vi "Lab Panel V2.2.vi"() -> ()   [LabVIEW 2013]
uses:
  <vilib>/Platform/TimedLoop/XDataNode/timing_clust.ctl
  <vilib>/Platform/TimedLoop/XDataNode/nitl_modes.ctl
  <vilib>/Platform/TimedLoop/XDataNode/wakeup.ctl
  <vilib>/platform/TimedLoop/XDataNode/XDataNode.xnode
  <vilib>/Platform/TimedLoop/XDataNode/XDNodeRunTimeDep.lvlib
panel:
  out "TEMP update":bool
  out "AI update":bool
  in  "stop":bool
  in  "Tab Control 2":T1(tab)
  out "LAB05-2 (SIG)":T2 {"PF" format="%.2f"; "AMPS" format="%.1f"}
  out "LAB05-1 (SIG)":T2 {"PF" format="%.2f"; "AMPS" format="%.1f"}
  out "LAB04-2 (SIG)":T2 {"PF" format="%.2f"; "AMPS" format="%.1f"}
  out "LAB04-1 (SIG)":T2 {"PF" format="%.2f"; "AMPS" format="%.1f"}
  out "LAB03-2 (SIG)":T2 {"PF" format="%.2f"; "AMPS" format="%.1f"}
  out "LAB03-1 (SIG)":T2 {"PF" format="%.2f"; "AMPS" format="%.1f"}
  out "LAB02-2 (SIG)":T2 {"PF" format="%.2f"; "AMPS" format="%.1f"}
  in  "LAB01-1RUN":bool
  in  "LAB05-1 (O/I)":bool
  in  "LAB05-2 (O/I)":bool
  in  "LAB04-1 (O/I)":bool
  in  "LAB04-2 (O/I)":bool
  in  "LAB02-1 (O/I)":bool
  in  "LAB02-2 (O/I)":bool
  in  "LAB01-2 (O/I)":bool
  in  "LAB01-1 (O/I)":bool
  in  "LAB03-1 (O/I)":bool
  in  "LAB05-2 RUN":bool
  in  "LAB05-1 RUN":bool
  in  "LAB04-2 RUN":bool
  in  "LAB04-1 RUN":bool
  in  "LAB03-2 RUN":bool
  in  "LAB03-1 RUN":bool
  in  "LAB02-2 RUN":bool
  in  "LAB02-1 RUN":bool
  in  "LAB01-2 RUN":bool
  in  "LAB05-2 SELECT":T3(radio)
  in  "LAB05-1 SELECT":T3(radio)
  in  "LAB04-2 SELECT":T3(radio)
  in  "LAB04-1 SELECT":T3(radio)
  in  "LAB03-2 SELECT":T3(radio)
  in  "LAB03-1 SELECT":T3(radio)
  in  "LAB02-2 SELECT":T3(radio)
  in  "LAB02-1 SELECT":T3(radio)
  in  "LAB01-2 SELECT":T3(radio)
  in  "LAB01-1 SELECT":T3(radio)
  in  "LAB03-2 (O/I)":bool
  out "LAB01-1 (SIG)":T2 {"PF" format="%.2f"; "AMPS" format="%.1f"}
  out "LAB01-2 (SIG)":T2 {"PF" format="%.2f"; "AMPS" format="%.1f"}
  out "LAB02-1 (SIG)":T2 {"PF" format="%.2f"; "AMPS" format="%.1f"}
  in  "LAB05 (SETTINGS 1)":T4={"1 Name"="", "1 Description"="", "1 (CYCLES)"=1.0, "1 (T-RISE mins)"=1.0, "1 (T-RISE deg C)"=1.0, "2 Name"="", "2 Description"="", "2 (CYCLES)"=1.0, "2 (T-RISE mins)"=1.0, "2 (T-RISE deg C)"=1.0} {"2 (T-RISE deg C)" min=1.0 max=100.0 step=1.0 format="%#.0f"; "2 (T-RISE mins)" min=0.0 max=1000.0 step=10.0 format="%#.0f"; "2 (CYCLES)" min=0.0 max=100000.0 step=10.0; "1 (T-RISE deg C)" min=1.0 max=100.0 step=1.0 format="%#.0f"; "1 (T-RISE mins)" min=0.0 max=1000.0 step=10.0 format="%#.0f"; "1 (CYCLES)" min=0.0 max=100000.0 step=10.0}
  in  "LAB04 (SETTINGS 1)":T4={"1 Name"="", "1 Description"="", "1 (CYCLES)"=1.0, "1 (T-RISE mins)"=1.0, "1 (T-RISE deg C)"=1.0, "2 Name"="", "2 Description"="", "2 (CYCLES)"=1.0, "2 (T-RISE mins)"=1.0, "2 (T-RISE deg C)"=1.0} {"2 (T-RISE deg C)" min=1.0 max=100.0 step=1.0 format="%#.0f"; "2 (T-RISE mins)" min=0.0 max=1000.0 step=10.0 format="%#.0f"; "2 (CYCLES)" min=0.0 max=100000.0 step=10.0; "1 (T-RISE deg C)" min=1.0 max=100.0 step=1.0 format="%#.0f"; "1 (T-RISE mins)" min=0.0 max=1000.0 step=10.0 format="%#.0f"; "1 (CYCLES)" min=0.0 max=100000.0 step=10.0}
  in  "LAB03 (SETTINGS 1)":T4={"1 Name"="", "1 Description"="", "1 (CYCLES)"=1.0, "1 (T-RISE mins)"=1.0, "1 (T-RISE deg C)"=1.0, "2 Name"="", "2 Description"="", "2 (CYCLES)"=1.0, "2 (T-RISE mins)"=1.0, "2 (T-RISE deg C)"=1.0} {"2 (T-RISE deg C)" min=1.0 max=100.0 step=1.0 format="%#.0f"; "2 (T-RISE mins)" min=0.0 max=1000.0 step=10.0 format="%#.0f"; "2 (CYCLES)" min=0.0 max=100000.0 step=10.0; "1 (T-RISE deg C)" min=1.0 max=100.0 step=1.0 format="%#.0f"; "1 (T-RISE mins)" min=0.0 max=1000.0 step=10.0 format="%#.0f"; "1 (CYCLES)" min=0.0 max=100000.0 step=10.0}
  out "LAB05 (DISP 1)":T5 {"2 (T-RISE min)" format="%#.0f"; "2 (CYCLE)" format="%#.0f"; "1 (T-RISE min)" format="%#.0f"; "1 (CYCLE)" format="%#.0f"}
  out "LAB04 (DISP 1)":T5 {"2 (T-RISE min)" format="%#.0f"; "2 (CYCLE)" format="%#.0f"; "1 (T-RISE min)" format="%#.0f"; "1 (CYCLE)" format="%#.0f"}
  out "LAB03 (DISP 1)":T5 {"2 (T-RISE min)" format="%#.0f"; "2 (CYCLE)" format="%#.0f"; "1 (T-RISE min)" format="%#.0f"; "1 (CYCLE)" format="%#.0f"}
  out "LAB02 (DISP 1)":T5 {"2 (T-RISE min)" format="%#.0f"; "2 (CYCLE)" format="%#.0f"; "1 (T-RISE min)" format="%#.0f"; "1 (CYCLE)" format="%#.0f"}
  in  "LAB02 (SETTINGS 1)":T4={"1 Name"="", "1 Description"="", "1 (CYCLES)"=1.0, "1 (T-RISE mins)"=1.0, "1 (T-RISE deg C)"=1.0, "2 Name"="", "2 Description"="", "2 (CYCLES)"=1.0, "2 (T-RISE mins)"=1.0, "2 (T-RISE deg C)"=1.0} {"2 (T-RISE deg C)" min=1.0 max=100.0 step=1.0 format="%#.0f"; "2 (T-RISE mins)" min=0.0 max=1000.0 step=10.0 format="%#.0f"; "2 (CYCLES)" min=0.0 max=100000.0 step=10.0; "1 (T-RISE deg C)" min=1.0 max=100.0 step=1.0 format="%#.0f"; "1 (T-RISE mins)" min=0.0 max=1000.0 step=10.0 format="%#.0f"; "1 (CYCLES)" min=0.0 max=100000.0 step=10.0}
  out "LAB01 (DISP 1)":T5 {"2 (T-RISE min)" format="%#.0f"; "2 (CYCLE)" format="%#.0f"; "1 (T-RISE min)" format="%#.0f"; "1 (CYCLE)" format="%#.0f"}
  in  "LAB01 (SETTINGS 1)":T4={"1 Name"="", "1 Description"="", "1 (CYCLES)"=1.0, "1 (T-RISE mins)"=1.0, "1 (T-RISE deg C)"=1.0, "2 Name"="", "2 Description"="", "2 (CYCLES)"=1.0, "2 (T-RISE mins)"=1.0, "2 (T-RISE deg C)"=1.0} {"2 (T-RISE deg C)" min=1.0 max=100.0 step=1.0 format="%#.0f"; "2 (T-RISE mins)" min=0.0 max=1000.0 step=10.0 format="%#.0f"; "2 (CYCLES)" min=0.0 max=100000.0 step=10.0; "1 (T-RISE deg C)" min=1.0 max=100.0 step=1.0 format="%#.0f"; "1 (T-RISE mins)" min=0.0 max=1000.0 step=10.0 format="%#.0f"; "1 (CYCLES)" min=0.0 max=100000.0 step=10.0}
  in  "JIG ON TIME (S)":dbl=1.0 min=1.0 max=10.0 step=0.5 format="%.1g"
  in  "JIG OFF TIME (S)":dbl=2.0 min=2.0 max=10.0 step=0.5 format="%.1g"
  out "LAB01-1 (JIG)":bool
  out "LAB01-2 (JIG)":bool
  out "LAB02-1 (JIG)":bool
  out "LAB02-2 (JIG)":bool
  out "LAB03-1 (JIG)":bool
  out "LAB03-2 (JIG)":bool
  out "LAB04-1 (JIG)":bool
  out "LAB04-2 (JIG)":bool
  out "LAB05-1 (JIG)":bool
  out "LAB05-2 (JIG)":bool
  in  "Tab Control":T6(tab)
  out "LAB01-2 (GRAPH)":dynamicdata(graph)
  out "LAB01-1 (GRAPH)":dynamicdata(graph)
  out "LAB02-2 (GRAPH)":dynamicdata(graph)
  out "LAB02-1 (GRAPH)":dynamicdata(graph)
  out "LAB03-2 (GRAPH)":dynamicdata(graph)
  out "LAB03-1 (GRAPH)":dynamicdata(graph)
  out "LAB04-2 (GRAPH)":dynamicdata(graph)
  out "LAB04-1 (GRAPH)":dynamicdata(graph)
  out "LAB05-2 (GRAPH)":dynamicdata(graph)
  out "LAB05-1 (GRAPH)":dynamicdata(graph)
  out "LAB05 TEMP":T7
  out "LAB04 TEMP":T7
  out "LAB02 TEMP":T7
  out "LAB01 TEMP":T7
  out "LAB03 TEMP":T7
  out "Analog Error Array":errorcluster[](array[cluster])
  out "AI loop time":dbl format="%.6g"
  out "loops":dbl
  in  "loop  delay(mS)":dbl
  out "on loops":dbl
  out "off loops":dbl
  out "jig cycle":dbl
  out "LAB01-1 (TDMS)":refnum<k34>
  out "LAB01-2 (TDMS)":refnum<k34>
  out "data file error":errorcluster
  out "LAB01 (CAL)":T8 {"2 (TN) cal" min=0.0 step=0.01 format="%.2f"; "2 (TL) cal" min=0.0 step=0.01 format="%.2f"; "2 (PF) cal" min=0.0 step=0.01 format="%.2f"; "2 (V) cal" min=0.0 step=0.01 format="%.2f"; "2 (A) cal" min=0.0 step=0.01 format="%.2f"; "1 (TN) cal" min=0.0 step=0.01 format="%.2f"; "1 (TL) cal" min=0.0 step=0.01 format="%.2f"; "1 (PF) cal" min=0.0 step=0.01 format="%.2f"; "1 (V) cal" min=0.0 step=0.01 format="%.2f"; "1  (A) cal" min=0.0 step=0.01 format="%.2f"}
  out "LAB03 (CAL)":T8 {"2 (TN) cal" min=0.0 step=0.01 format="%.2f"; "2 (TL) cal" min=0.0 step=0.01 format="%.2f"; "2 (PF) cal" min=0.0 step=0.01 format="%.2f"; "2 (V) cal" min=0.0 step=0.01 format="%.2f"; "2 (A) cal" min=0.0 step=0.01 format="%.2f"; "1 (TN) cal" min=0.0 step=0.01 format="%.2f"; "1 (TL) cal" min=0.0 step=0.01 format="%.2f"; "1 (PF) cal" min=0.0 step=0.01 format="%.2f"; "1 (V) cal" min=0.0 step=0.01 format="%.2f"; "1  (A) cal" min=0.0 step=0.01 format="%.2f"}
  out "LAB02 (CAL)":T9 {"2 (TN) cal" min=0.0 step=0.01 format="%.2f"; "2 (TL) cal" min=0.0 step=0.01 format="%.2f"; "2 (PF) cal" min=0.0 step=0.01 format="%.2f"; "2 (V) cal" min=0.0 step=0.01 format="%.2f"; "2 (A) cal" min=0.0 step=0.01 format="%.2f"; "1 (TN) cal" min=0.0 step=0.01 format="%.2f"; "1 (TL) cal" min=0.0 step=0.01 format="%.2f"; "1 (PF) cal" min=0.0 step=0.01 format="%.2f"; "1 (V) cal" min=0.0 step=0.01 format="%.2f"; "1 (A) cal" min=0.0 step=0.01 format="%.2f"}
  out "LAB05 (CAL)":T8 {"2 (TN) cal" min=0.0 step=0.01 format="%.2f"; "2 (TL) cal" min=0.0 step=0.01 format="%.2f"; "2 (PF) cal" min=0.0 step=0.01 format="%.2f"; "2 (V) cal" min=0.0 step=0.01 format="%.2f"; "2 (A) cal" min=0.0 step=0.01 format="%.2f"; "1 (TN) cal" min=0.0 step=0.01 format="%.2f"; "1 (TL) cal" min=0.0 step=0.01 format="%.2f"; "1 (PF) cal" min=0.0 step=0.01 format="%.2f"; "1 (V) cal" min=0.0 step=0.01 format="%.2f"; "1  (A) cal" min=0.0 step=0.01 format="%.2f"}
  out "LAB04 (CAL)":T8 {"2 (TN) cal" min=0.0 step=0.01 format="%.2f"; "2 (TL) cal" min=0.0 step=0.01 format="%.2f"; "2 (PF) cal" min=0.0 step=0.01 format="%.2f"; "2 (V) cal" min=0.0 step=0.01 format="%.2f"; "2 (A) cal" min=0.0 step=0.01 format="%.2f"; "1 (TN) cal" min=0.0 step=0.01 format="%.2f"; "1 (TL) cal" min=0.0 step=0.01 format="%.2f"; "1 (PF) cal" min=0.0 step=0.01 format="%.2f"; "1 (V) cal" min=0.0 step=0.01 format="%.2f"; "1  (A) cal" min=0.0 step=0.01 format="%.2f"}
  out "calibration file error out":errorcluster
  in  "CALIBRATE":bool
  # "LAB01"
  # "LAB02"
  # "LAB05"
  # "LAB03"
  # "LAB04"
  # "LAB01"
  # "LAB02"
  # "LAB03"
  # "LAB04"
  # "LAB05"
  # "JIG SET"
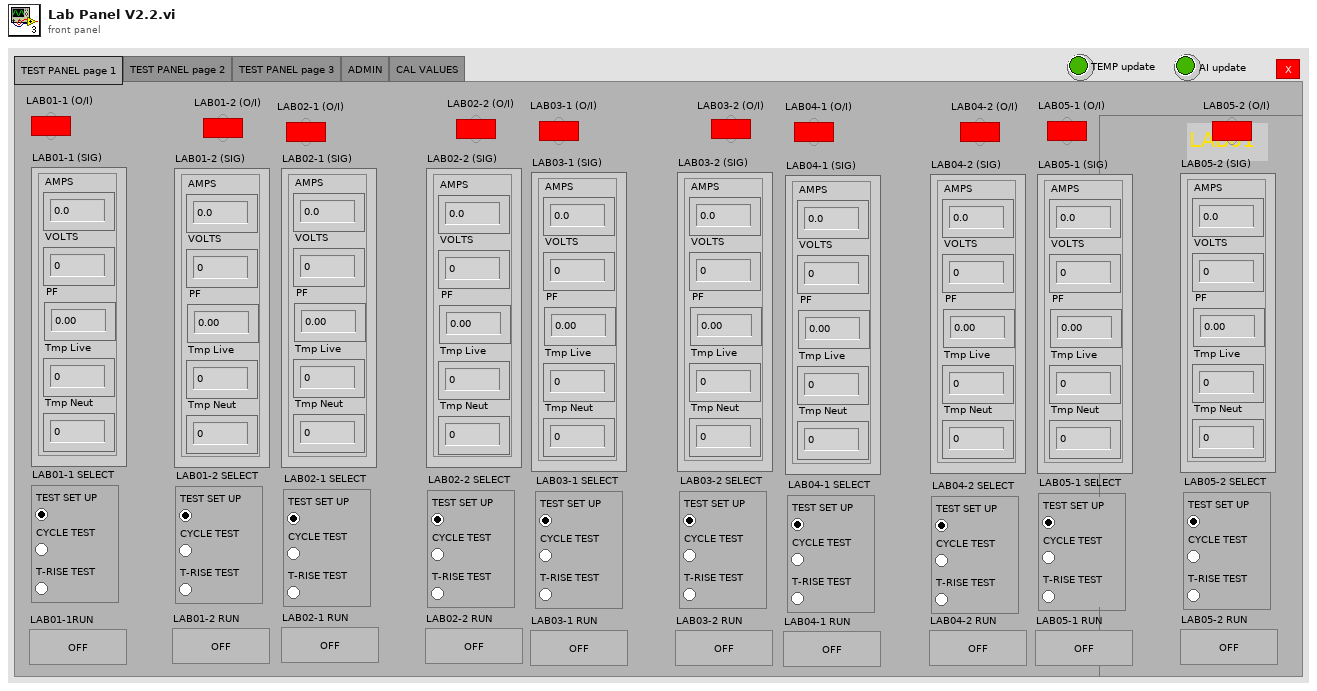
[diagram p1: front panel]
types:
  T1 = enum32{"TEST PANEL page 1", "TEST PANEL page 2", "TEST PANEL page 3", "ADMIN", "CAL VALUES"}
  T2 = cluster{"AMPS":dbl, "VOLTS":dbl, "PF":dbl, "Tmp Live":dbl, "Tmp Neut":dbl}
  T3 = enum32{"TEST SET UP", "CYCLE TEST", "T-RISE TEST"}
  T4 = cluster{"1 Name":string, "1 Description":string, "1 (CYCLES)":dbl, "1 (T-RISE mins)":dbl, "1 (T-RISE deg C)":dbl, "2 Name":string, "2 Description":string, "2 (CYCLES)":dbl, "2 (T-RISE mins)":dbl, "2 (T-RISE deg C)":dbl}
  T5 = cluster{"1 (CYCLE)":dbl, "1 (T-RISE min)":dbl, "1 (STATUS)":string, "2 (CYCLE)":dbl, "2 (T-RISE min)":dbl, "2 (STATUS)":string}
  T6 = enum32{"LAB01", "LAB02", "LAB03", "LAB04", "LAB05", "TEMPERATURE", "ERROR"}
  T7 = cluster{"T1 Live":dbl, "T1 Neut":dbl, "T2 Live":dbl, "T2 Neut":dbl, "ID":dbl, "ER":dbl}
  T8 = cluster{"1  (A) cal":dbl, "1 (V) cal":dbl, "1 (PF) cal":dbl, "1 (TL) cal":dbl, "1 (TN) cal":dbl, "2 (A) cal":dbl, "2 (V) cal":dbl, "2 (PF) cal":dbl, "2 (TL) cal":dbl, "2 (TN) cal":dbl}
  T9 = cluster{"1 (A) cal":dbl, "1 (V) cal":dbl, "1 (PF) cal":dbl, "1 (TL) cal":dbl, "1 (TN) cal":dbl, "2 (A) cal":dbl, "2 (V) cal":dbl, "2 (PF) cal":dbl, "2 (TL) cal":dbl, "2 (TN) cal":dbl}
  T10 = typedef "XDNodeRunTimeDep.lvlib/timing_clust.ctl" = cluster{"Expected End [f-1]":u64, "Actual End [f-1]":u64, "Finished Late? [f-1]":bool, "Expected End [i-1]":u64, "Actual End [i-1]":u64, "Finished Late? [i-1]":bool, "Expected Start [i]":u64, "Actual Start [i]":u64, "Expected Start [f]":u64, "Actual Start [f]":u64, "Source Name":string, "Structure Name":string, "Period":i64, "Deadline":i64, "Offset":i64, "Start":i64, "Priority":i32, "Timeout":i32, "Mode":T11, "Wakeup Reason":T12, "Error":errorcluster, "Source Type":string, "Secondary Source Type":string, "Global End Time":u64, "Global Start Time":u64, "Frame Duration":u64, "Iteration Duration":u64, "Assigned CPU":i32, "I/O Scan Engine Mode":u32}
  T11 = typedef "XDNodeRunTimeDep.lvlib/nitl_modes.ctl" = enum32{"No Change", "Process missed periods, maintain original phase", "Discard missed periods, maintain original phase", "Process missed periods, ignore original phase", "Discard missed periods, ignore original phase"}
  T12 = typedef "XDNodeRunTimeDep.lvlib/wakeup.ctl" = enum32{"Normal", "Aborted", "Asynchronous wakeup", "Timing source error", "Timed loop error", "Timeout"}
  T13 = enum16{"open", "open or create", "create or replace", "create", "open (read-only)"}
  T14 = cluster{"T1":dbl, "T2":dbl, "T3":dbl, "T4":dbl, "ID":dbl, "ER":dbl}
  T15 = cluster{"LAB01-1 (A)":dbl, "LAB01-1 (V)":dbl, "LAB01-1 (PF)":dbl, "LAB01-2 (A)":dbl, "LAB01-2 (V)":dbl, "LAB01-2 (PF)":dbl}
  T16 = cluster{"LAB02-1 (A)":dbl, "LAB02-1 (V)":dbl, "LAB02-1 (PF)":dbl, "LAB02-2 (A)":dbl, "LAB02-2 (V)":dbl, "LAB02-2 (PF)":dbl}
  T17 = cluster{"LAB03-1 (A)":dbl, "LAB03-1 (V)":dbl, "LAB03-1 (PF)":dbl, "LAB03-2 (A)":dbl, "LAB03-2 (V)":dbl, "LAB03-2 (PF)":dbl}
  T18 = cluster{"LAB04-1 (A)":dbl, "LAB04-1 (V)":dbl, "LAB04-1 (PF)":dbl, "LAB04-2 (A)":dbl, "LAB04-2 (V)":dbl, "LAB04-2 (PF)":dbl}
  T19 = cluster{"LAB05-1 (A)":dbl, "LAB05-1 (V)":dbl, "LAB05-1 (PF)":dbl, "LAB05-2 (A)":dbl, "LAB05-2 (V)":dbl, "LAB05-2 (PF)":dbl}
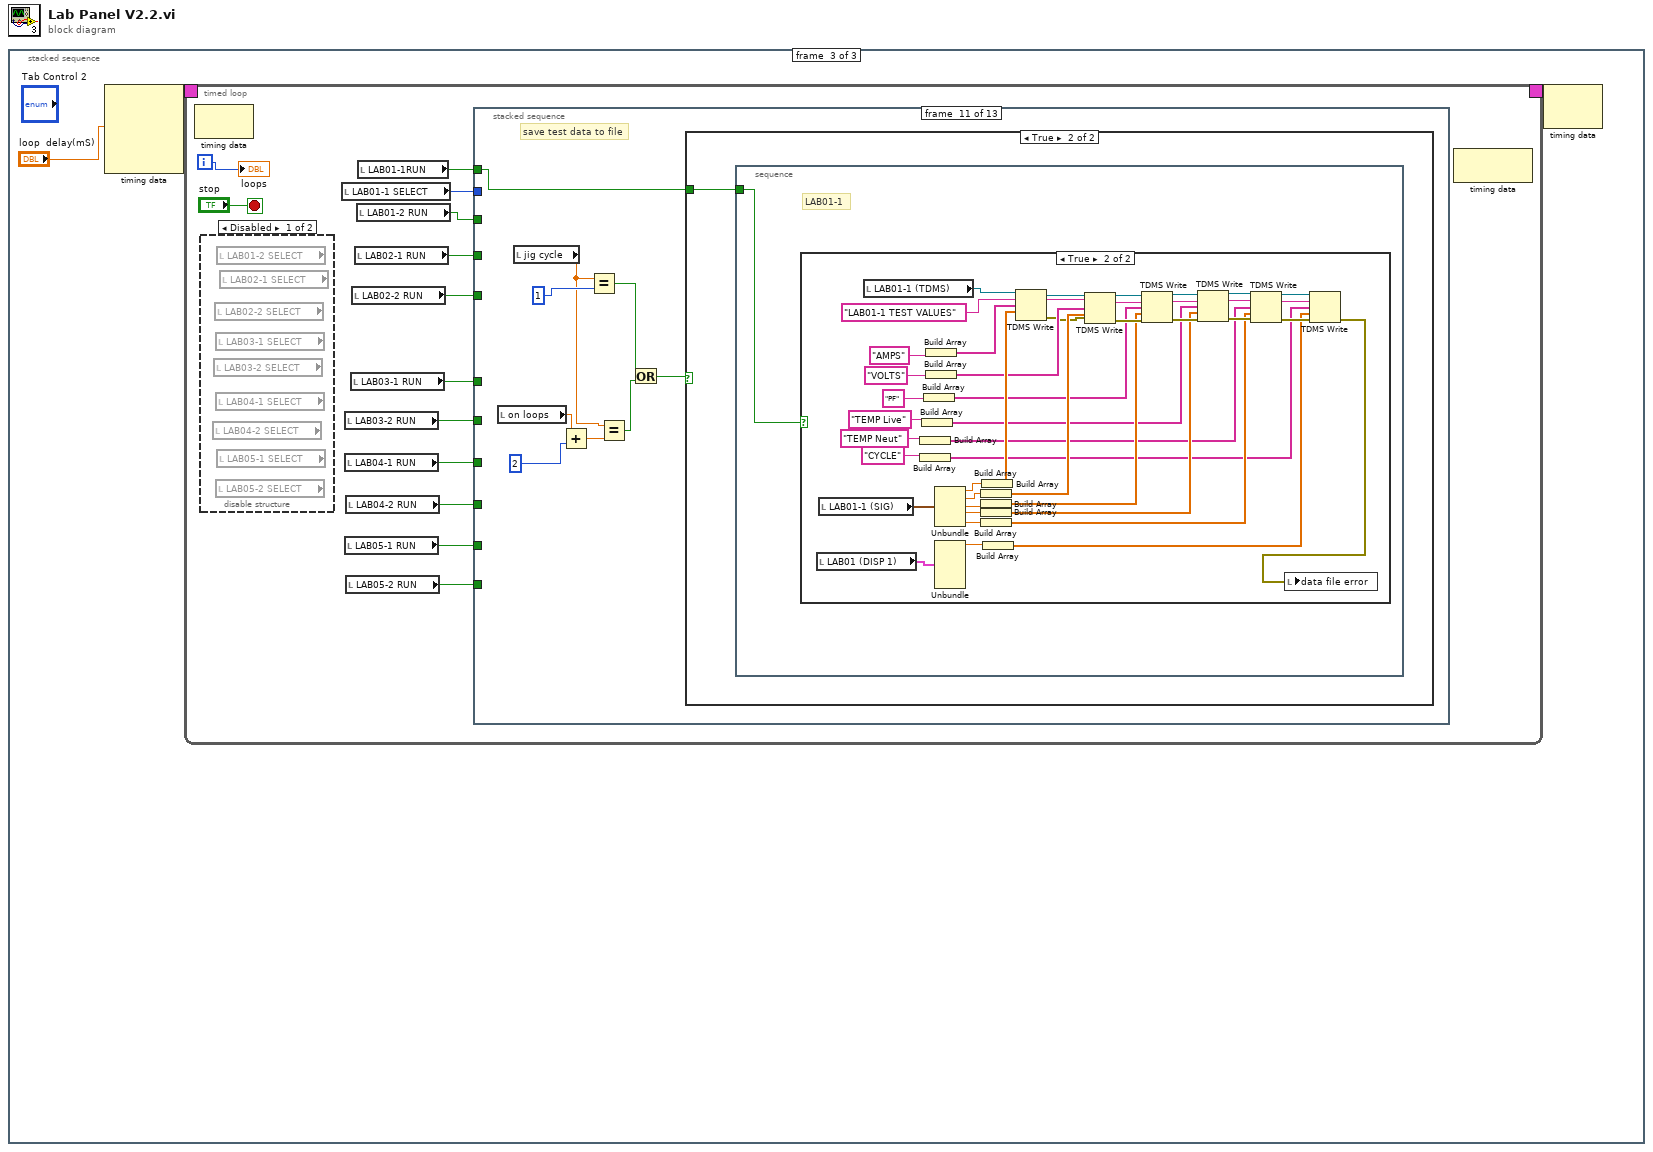
[diagram p0: block diagram]
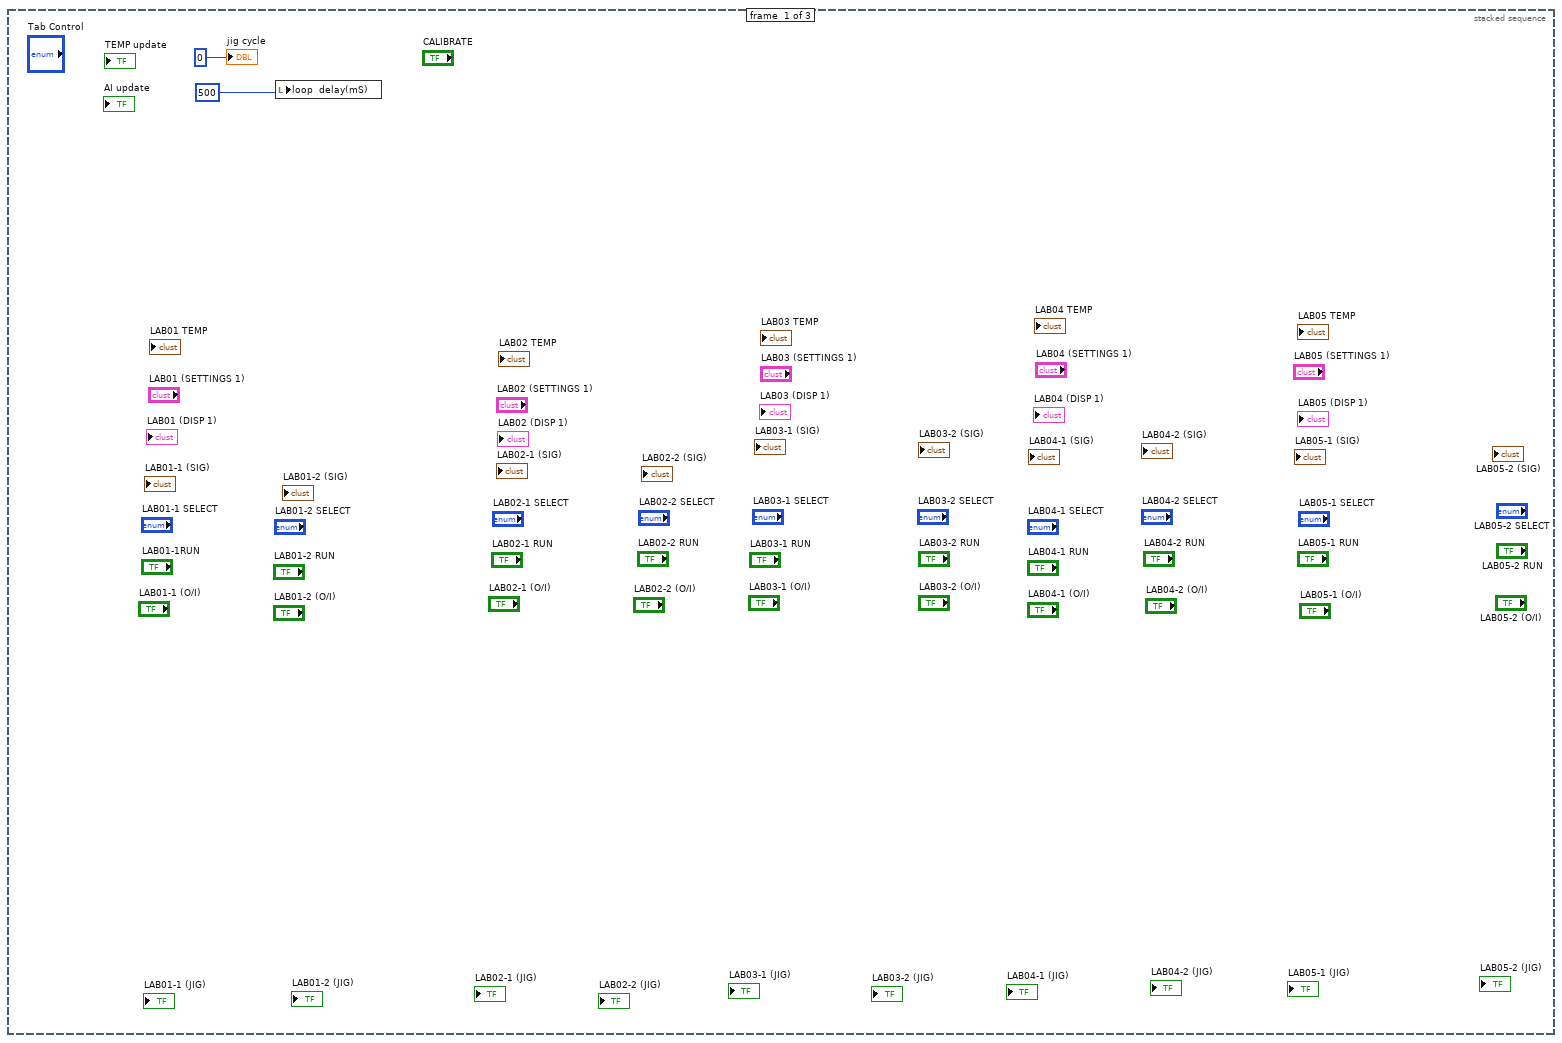
[diagram p2: hidden frame]
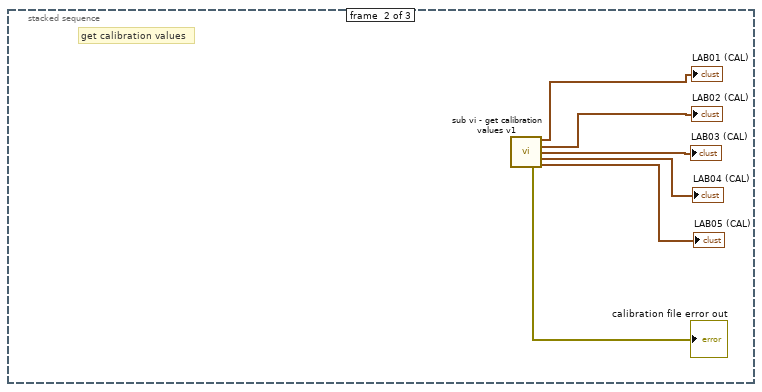
[diagram p3: hidden frame]
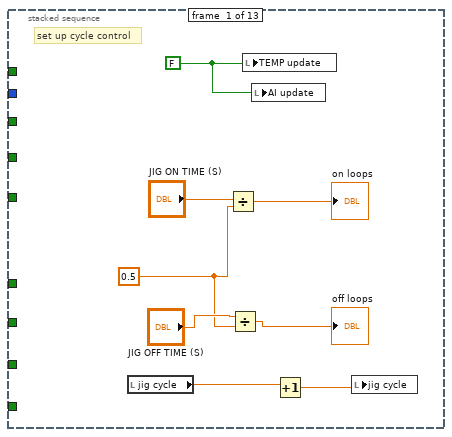
[diagram p5: hidden frame]
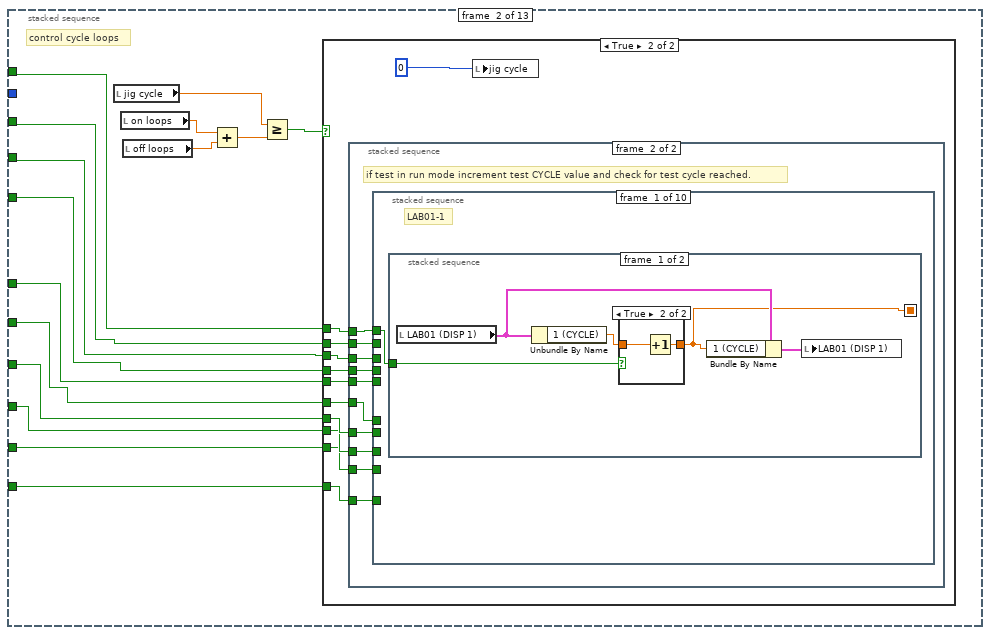
[diagram p6: hidden frame]
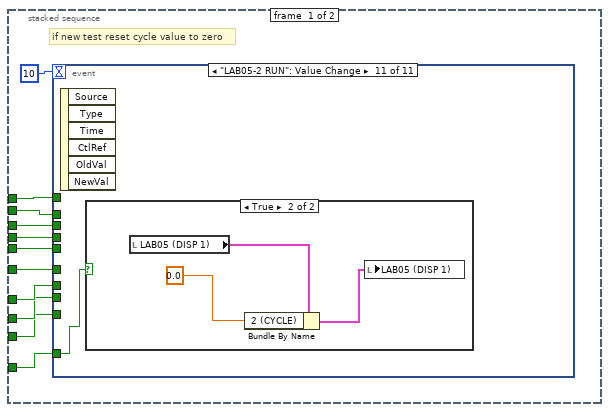
[diagram p8: hidden frame]
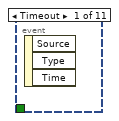
[diagram p9: hidden frame]
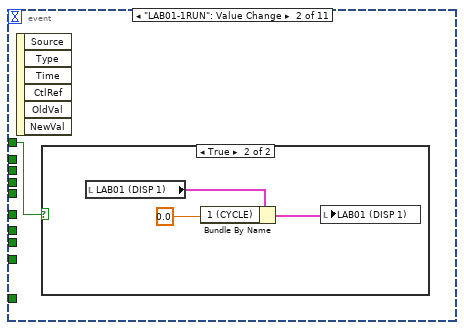
[diagram p10: hidden frame]
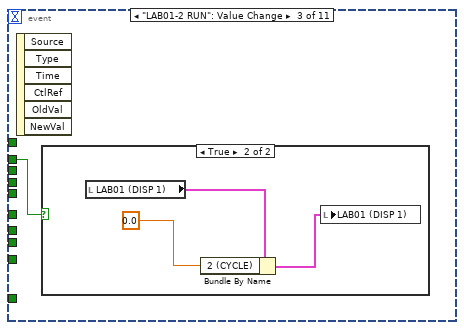
[diagram p12: hidden frame]
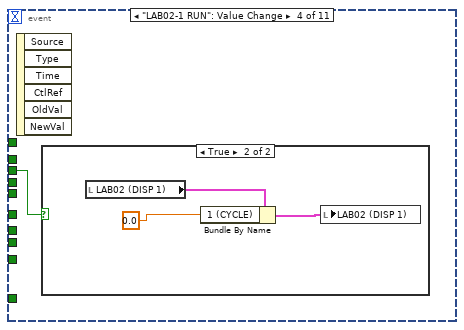
[diagram p14: hidden frame]
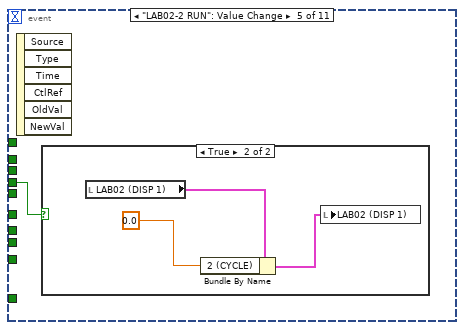
[diagram p16: hidden frame]
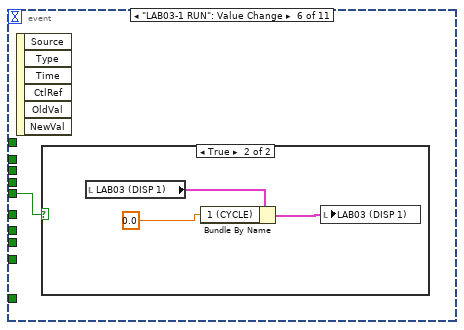
[diagram p18: hidden frame]
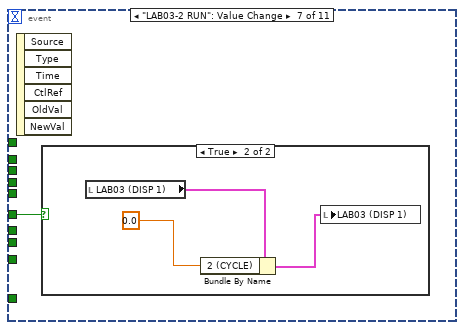
[diagram p20: hidden frame]
diagram:
  n1 = stacked-sequence {
    frame #0 {
      n2 = local write "loop  delay(mS)"(500) -> ()
      "jig cycle" <- 0
    }
    frame #1 {
      # "get calibration values"
      n3 = call "sub vi - get calibration values v1.vi"() -> ("LAB01 (CAL)"=→"LAB01 (CAL)":T8, "LAB02 (CAL)"=→"LAB02 (CAL)":T9, "LAB03 (CAL)"=→"LAB03 (CAL)":T8, "LAB04 (CAL)"=→"LAB04 (CAL)":T8, "calibration file error out"=→"calibration file error out":errorcluster, "LAB05 (CAL)"=→"LAB05 (CAL)":T8)  [unwired: 10 in]
    }
    frame #2 {
      n4 = node-c288("loop  delay(mS)") -> (w11:T10)  [unwired: 3 in]
      n5 = timed-loop {
        timing: w11 -> [_]
        timing-out: [_] -> w10
        i -> [w24]
        stop <- "stop" stop-if-true
        n6 = node-c288() -> ()  [unwired: 1 in, 1 out]
        n7 = disable-structure shown="Disabled" {
          frame Disabled {
            n8 = local read "LAB04-2 SELECT"() -> ()  [unwired: 1 out]
            n9 = local read "LAB03-2 SELECT"() -> ()  [unwired: 1 out]
            n10 = local read "LAB02-2 SELECT"() -> ()  [unwired: 1 out]
            n11 = local read "LAB03-1 SELECT"() -> ()  [unwired: 1 out]
            n12 = local read "LAB04-1 SELECT"() -> ()  [unwired: 1 out]
            n13 = local read "LAB05-2 SELECT"() -> ()  [unwired: 1 out]
            n14 = local read "LAB01-2 SELECT"() -> ()  [unwired: 1 out]
            n15 = local read "LAB05-1 SELECT"() -> ()  [unwired: 1 out]
            n16 = local read "LAB02-1 SELECT"() -> ()  [unwired: 1 out]
          }
          frame Enabled {
          }
        }
        n17 = local read "LAB01-1 SELECT"() -> (w12:T3)
        n18 = local read "LAB03-2 RUN"() -> (w17:bool)
        n19 = local read "LAB04-1 RUN"() -> (w16:bool)
        n20 = local read "LAB05-1 RUN"() -> (w14:bool)
        n21 = local read "LAB04-2 RUN"() -> (w15:bool)
        n22 = local read "LAB05-2 RUN"() -> (w13:bool)
        n23 = local read "LAB03-1 RUN"() -> (w18:bool)
        n24 = local read "LAB02-2 RUN"() -> (w19:bool)
        n25 = local read "LAB02-1 RUN"() -> (w20:bool)
        n26 = local read "LAB01-2 RUN"() -> (w21:bool)
        n27 = local read "LAB01-1RUN"() -> (w22:bool)
        n28 = stacked-sequence {
          tunnel: w22 -> [_ w44 w336 _ w411 w466 _ _ _ _ w833 _ _]
          tunnel: w21 -> [_ w43 w335 _ _ _ _ _ _ _ _ _ _]
          tunnel: w20 -> [_ w42 w334 _ _ _ _ _ _ _ _ _ _]
          tunnel: w19 -> [_ w41 w333 _ _ _ _ _ _ _ _ _ _]
          tunnel: w18 -> [_ w40 w332 _ _ _ _ _ _ _ _ _ _]
          tunnel: w17 -> [_ w39 w331 _ _ _ _ _ _ _ _ _ _]
          tunnel: w16 -> [_ w38 w330 _ _ _ _ _ _ _ _ _ _]
          tunnel: w15 -> [_ w37 w329 _ _ _ _ _ _ _ _ _ _]
          tunnel: w14 -> [_ w36 w328 _ _ _ _ _ _ _ _ _ _]
          tunnel: w13 -> [_ w35 w327 _ _ _ _ _ _ _ _ _ _]
          tunnel: w12 -> [_ _ _ _ w412 _ _ _ _ _ _ _ _]
          frame #0 {
            w27 = FALSE
            w32 = 0.5
            # "set up cycle control"
            n29 = local read "jig cycle"() -> (w31:dbl)
            n30 = Divide(x="JIG ON TIME (S)", y=w32) -> (x/y=→"on loops":dbl)
            n31 = Divide(x="JIG OFF TIME (S)", y=w32) -> (x/y=→"off loops":dbl)
            n32 = local write "TEMP update"(w27) -> ()
            n33 = local write "AI update"(w27) -> ()
            n34 = Increment(x=w31) -> (x+1=w30:dbl)
            n35 = local write "jig cycle"(w30) -> ()
          }
          frame #1 {
            # "control cycle loops"
            n36 = local read "jig cycle"() -> (w46:dbl)
            n37 = local read "on loops"() -> (w49:dbl)
            n38 = local read "off loops"() -> (w48:dbl)
            n39 = Add(x=w49, y=w48) -> (x+y=w47:dbl)
            n40 = Greater Or Equal?(x=w46, y=w47) -> (x >= y?=w45:bool)
            n41 = case shown="True" w45 {
              tunnel: w44 -> [_ w59]
              tunnel: w43 -> [_ w58]
              tunnel: w42 -> [_ w57]
              tunnel: w41 -> [_ w56]
              tunnel: w40 -> [_ w55]
              tunnel: w39 -> [_ w54]
              tunnel: w38 -> [_ w53]
              tunnel: w37 -> [_ w52]
              tunnel: w36 -> [_ w51]
              tunnel: w35 -> [_ w50]
              frame False {
              }
              frame True {
                n42 = stacked-sequence {
                  tunnel: w59 -> [w70 w121]
                  tunnel: w58 -> [w69 w120]
                  tunnel: w57 -> [w68 w119]
                  tunnel: w56 -> [w67 w118]
                  tunnel: w55 -> [w66 w117]
                  tunnel: w54 -> [w65 w116]
                  tunnel: w53 -> [w64 w115]
                  tunnel: w52 -> [w63 w114]
                  tunnel: w51 -> [w62 w113]
                  tunnel: w50 -> [w61 w112]
                  frame #0 {
                    # "if new test reset cycle value to zero"
                    n43 = event shown="[10] \"LAB05-2 RUN\": Value Change" {
                      selector: _ -> [_ _ _ _ _ _ _ _ _ _ _]
                      dyn-events: _ -> [_ _ _ _ _ _ _ _ _ _ _]
                      timeout: 10 -> [_ _ _ _ _ _ _ _ _ _ _]
                      tunnel: w70 -> [_ w72 _ _ _ _ _ _ _ _ _]
                      tunnel: w69 -> [_ _ w76 _ _ _ _ _ _ _ _]
                      tunnel: w68 -> [_ _ _ w80 _ _ _ _ _ _ _]
                      tunnel: w67 -> [_ _ _ _ w84 _ _ _ _ _ _]
                      tunnel: w66 -> [_ _ _ _ _ w88 _ _ _ _ _]
                      tunnel: w65 -> [_ _ _ _ _ _ w92 _ _ _ _]
                      tunnel: w64 -> [_ _ _ _ _ _ _ w96 _ _ _]
                      tunnel: w63 -> [_ _ _ _ _ _ _ _ w100 _ _]
                      tunnel: w62 -> [_ _ _ _ _ _ _ _ _ w104 _]
                      tunnel: w61 -> [_ _ _ _ _ _ _ _ _ _ w108]
                      event Timeout {
                        n44 = event-data() -> ()  [unwired: 1 in, 3 out]
                      }
                      event "LAB01-1RUN": Value Change {
                        n45 = event-data() -> ()  [unwired: 1 in, 6 out]
                        n46 = case shown="True" w72 {
                          frame False {
                          }
                          frame True {
                            n47 = local read "LAB01 (DISP 1)"() -> (w75:T5)
                            n48 = Bundle By Name(cluster=w75, "1 (CYCLE)"=0.0) -> (w73:T5)
                            n49 = local write "LAB01 (DISP 1)"(w73) -> ()
                          }
                        }
                      }
                      event "LAB01-2 RUN": Value Change {
                        n50 = event-data() -> ()  [unwired: 1 in, 6 out]
                        n51 = case shown="True" w76 {
                          frame False {
                          }
                          frame True {
                            n52 = local read "LAB01 (DISP 1)"() -> (w79:T5)
                            n53 = Bundle By Name(cluster=w79, "2 (CYCLE)"=0.0) -> (w78:T5)
                            n54 = local write "LAB01 (DISP 1)"(w78) -> ()
                          }
                        }
                      }
                      event "LAB02-1 RUN": Value Change {
                        n55 = event-data() -> ()  [unwired: 1 in, 6 out]
                        n56 = case shown="True" w80 {
                          frame False {
                          }
                          frame True {
                            n57 = local read "LAB02 (DISP 1)"() -> (w83:T5)
                            n58 = Bundle By Name(cluster=w83, "1 (CYCLE)"=0.0) -> (w82:T5)
                            n59 = local write "LAB02 (DISP 1)"(w82) -> ()
                          }
                        }
                      }
                      event "LAB02-2 RUN": Value Change {
                        n60 = event-data() -> ()  [unwired: 1 in, 6 out]
                        n61 = case shown="True" w84 {
                          frame False {
                          }
                          frame True {
                            n62 = local read "LAB02 (DISP 1)"() -> (w87:T5)
                            n63 = Bundle By Name(cluster=w87, "2 (CYCLE)"=0.0) -> (w86:T5)
                            n64 = local write "LAB02 (DISP 1)"(w86) -> ()
                          }
                        }
                      }
                      event "LAB03-1 RUN": Value Change {
                        n65 = event-data() -> ()  [unwired: 1 in, 6 out]
                        n66 = case shown="True" w88 {
                          frame False {
                          }
                          frame True {
                            n67 = local read "LAB03 (DISP 1)"() -> (w91:T5)
                            n68 = Bundle By Name(cluster=w91, "1 (CYCLE)"=0.0) -> (w90:T5)
                            n69 = local write "LAB03 (DISP 1)"(w90) -> ()
                          }
                        }
                      }
                      event "LAB03-2 RUN": Value Change {
                        n70 = event-data() -> ()  [unwired: 1 in, 6 out]
                        n71 = case shown="True" w92 {
                          frame False {
                          }
                          frame True {
                            n72 = local read "LAB03 (DISP 1)"() -> (w95:T5)
                            n73 = Bundle By Name(cluster=w95, "2 (CYCLE)"=0.0) -> (w94:T5)
                            n74 = local write "LAB03 (DISP 1)"(w94) -> ()
                          }
                        }
                      }
                      event "LAB04-1 RUN": Value Change {
                        n75 = event-data() -> ()  [unwired: 1 in, 6 out]
                        n76 = case shown="True" w96 {
                          frame False {
                          }
                          frame True {
                            n77 = local read "LAB04 (DISP 1)"() -> (w99:T5)
                            n78 = Bundle By Name(cluster=w99, "1 (CYCLE)"=0.0) -> (w98:T5)
                            n79 = local write "LAB04 (DISP 1)"(w98) -> ()
                          }
                        }
                      }
                      event "LAB04-2 RUN": Value Change {
                        n80 = event-data() -> ()  [unwired: 1 in, 6 out]
                        n81 = case shown="True" w100 {
                          frame False {
                          }
                          frame True {
                            n82 = local read "LAB04 (DISP 1)"() -> (w103:T5)
                            n83 = Bundle By Name(cluster=w103, "2 (CYCLE)"=0.0) -> (w102:T5)
                            n84 = local write "LAB04 (DISP 1)"(w102) -> ()
                          }
                        }
                      }
                      event "LAB05-1 RUN": Value Change {
                        n85 = event-data() -> ()  [unwired: 1 in, 6 out]
                        n86 = case shown="True" w104 {
                          frame False {
                          }
                          frame True {
                            n87 = local read "LAB05 (DISP 1)"() -> (w107:T5)
                            n88 = Bundle By Name(cluster=w107, "1 (CYCLE)"=0.0) -> (w106:T5)
                            n89 = local write "LAB05 (DISP 1)"(w106) -> ()
                          }
                        }
                      }
                      event "LAB05-2 RUN": Value Change {
                        n90 = event-data() -> ()  [unwired: 1 in, 6 out]
                        n91 = case shown="True" w108 {
                          frame False {
                          }
                          frame True {
                            n92 = local read "LAB05 (DISP 1)"() -> (w111:T5)
                            n93 = Bundle By Name(cluster=w111, "2 (CYCLE)"=0.0) -> (w110:T5)
                            n94 = local write "LAB05 (DISP 1)"(w110) -> ()
                          }
                        }
                      }
                    }
                  }
                  frame #1 {
                    # "if test in run mode increment test CYCLE value and check for test cycle reached."
                    n95 = stacked-sequence {
                      tunnel: w121 -> [w122 w139 w157 w176 w196 w217 w239 w262 w286 w311]
                      tunnel: w120 -> [_ w138 w156 w175 w195 w216 w238 w261 w285 w310]
                      tunnel: w119 -> [_ _ w155 w174 w194 w215 w237 w260 w284 w309]
                      tunnel: w118 -> [_ _ _ w173 w193 w214 w236 w259 w283 w308]
                      tunnel: w117 -> [_ _ _ _ w192 w213 w235 w258 w282 w307]
                      tunnel: w116 -> [_ _ _ _ _ w212 w234 w257 w281 w306]
                      tunnel: w115 -> [_ _ _ _ _ _ w233 w256 w280 w305]
                      tunnel: w114 -> [_ _ _ _ _ _ _ w255 w279 w304]
                      tunnel: w113 -> [_ _ _ _ _ _ _ _ w278 w303]
                      tunnel: w112 -> [_ _ _ _ _ _ _ _ _ w302]
                      frame #0 {
                        # "LAB01-1"
                        n96 = stacked-sequence {
                          seq-local: [w123 _] -> [_ w135]
                          tunnel: w122 -> [w127 w133]
                          frame #0 {
                            n97 = local read "LAB01 (DISP 1)"() -> (w124:T5)
                            n98 = Unbundle By Name(w124) -> ("1 (CYCLE)"=w125:dbl)
                            n99 = case shown="True" w127 {
                              tunnel: w125 -> [w128 w130]
                              tunnel: [w128 w129] -> w123
                              frame False {
                              }
                              frame True {
                                n100 = Increment(x=w130) -> (x+1=w129:dbl)
                              }
                            }
                            n101 = Bundle By Name(cluster=w124, "1 (CYCLE)"=w123) -> (w126:T5)
                            n102 = local write "LAB01 (DISP 1)"(w126) -> ()
                          }
                          frame #1 {
                            # "stop test if test cycles reached"
                            n103 = local read "LAB01 (SETTINGS 1)"() -> (w137:T4)
                            n104 = Unbundle By Name(w137) -> ("1 (CYCLES)"=w136:dbl)
                            n105 = Greater Or Equal?(x=w135, y=w136) -> (x >= y?=w134:bool)
                            n106 = Select(t=FALSE, s=w134, f=w133) -> (s? t:f=w131:bool)
                            n107 = local write "LAB01-1RUN"(w131) -> ()
                          }
                        }
                      }
                      frame #1 {
                        # "LAB01-2"
                        n108 = stacked-sequence {
                          seq-local: [w141 _] -> [_ w154]
                          tunnel: w139 -> [_ _]
                          tunnel: w138 -> [w140 w148]
                          frame #0 {
                            # "update cycle value"
                            n109 = local read "LAB01 (DISP 1)"() -> (w143:T5)
                            n110 = Unbundle By Name(w143) -> ("2 (CYCLE)"=w142:dbl)
                            n111 = case shown="True" w140 {
                              tunnel: w142 -> [w145 w147]
                              tunnel: [w145 w146] -> w141
                              frame False {
                              }
                              frame True {
                                n112 = Increment(x=w147) -> (x+1=w146:dbl)
                              }
                            }
                            n113 = Bundle By Name(cluster=w143, "2 (CYCLE)"=w141) -> (w144:T5)
                            n114 = local write "LAB01 (DISP 1)"(w144) -> ()
                          }
                          frame #1 {
                            # "stop test if test cycles reached"
                            n115 = local read "LAB01 (SETTINGS 1)"() -> (w150:T4)
                            n116 = Unbundle By Name(w150) -> ("2 (CYCLES)"=w149:dbl)
                            n117 = Greater Or Equal?(x=w154, y=w149) -> (x >= y?=w153:bool)
                            n118 = Select(t=FALSE, s=w153, f=w148) -> (s? t:f=w151:bool)
                            n119 = local write "LAB01-2 RUN"(w151) -> ()
                          }
                        }
                      }
                      frame #2 {
                        # "LAB02-1"
                        n120 = stacked-sequence {
                          seq-local: [w159 _] -> [_ w172]
                          tunnel: w157 -> [_ _]
                          tunnel: w156 -> [_ _]
                          tunnel: w155 -> [w160 w167]
                          frame #0 {
                            # "update cycle value"
                            n121 = local read "LAB02 (DISP 1)"() -> (w161:T5)
                            n122 = Unbundle By Name(w161) -> ("1 (CYCLE)"=w158:dbl)
                            n123 = case shown="True" w160 {
                              tunnel: [w163 w165] -> w159
                              tunnel: w158 -> [w163 w164]
                              frame False {
                              }
                              frame True {
                                n124 = Increment(x=w164) -> (x+1=w165:dbl)
                              }
                            }
                            n125 = Bundle By Name(cluster=w161, "1 (CYCLE)"=w159) -> (w162:T5)
                            n126 = local write "LAB02 (DISP 1)"(w162) -> ()
                          }
                          frame #1 {
                            # "stop test if test cycles reached"
                            n127 = local read "LAB02 (SETTINGS 1)"() -> (w168:T4)
                            n128 = Unbundle By Name(w168) -> ("1 (CYCLES)"=w166:dbl)
                            n129 = Greater Or Equal?(x=w172, y=w166) -> (x >= y?=w171:bool)
                            n130 = Select(t=FALSE, s=w171, f=w167) -> (s? t:f=w169:bool)
                            n131 = local write "LAB02-1 RUN"(w169) -> ()
                          }
                        }
                      }
                      frame #3 {
                        # "LAB02-2"
                        n132 = stacked-sequence {
                          seq-local: [w177 _] -> [_ w191]
                          tunnel: w176 -> [_ _]
                          tunnel: w175 -> [_ _]
                          tunnel: w174 -> [_ _]
                          tunnel: w173 -> [w179 w185]
                          frame #0 {
                            # "update cycle value"
                            n133 = local read "LAB02 (DISP 1)"() -> (w180:T5)
                            n134 = Unbundle By Name(w180) -> ("2 (CYCLE)"=w178:dbl)
                            n135 = case shown="True" w179 {
                              tunnel: [w182 w184] -> w177
                              tunnel: w178 -> [w182 w183]
                              frame False {
                              }
                              frame True {
                                n136 = Increment(x=w183) -> (x+1=w184:dbl)
                              }
                            }
                            n137 = Bundle By Name(cluster=w180, "2 (CYCLE)"=w177) -> (w181:T5)
                            n138 = local write "LAB02 (DISP 1)"(w181) -> ()
                          }
                          frame #1 {
                            # "stop test if test cycles reached"
                            n139 = local read "LAB02 (SETTINGS 1)"() -> (w187:T4)
                            n140 = Unbundle By Name(w187) -> ("2 (CYCLES)"=w186:dbl)
                            n141 = Greater Or Equal?(x=w191, y=w186) -> (x >= y?=w190:bool)
                            n142 = Select(t=FALSE, s=w190, f=w185) -> (s? t:f=w188:bool)
                            n143 = local write "LAB02-2 RUN"(w188) -> ()
                          }
                        }
                      }
                      frame #4 {
                        # "LAB03-1"
                        n144 = stacked-sequence {
                          seq-local: [w197 _] -> [_ w211]
                          tunnel: w196 -> [_ _]
                          tunnel: w195 -> [_ _]
                          tunnel: w194 -> [_ _]
                          tunnel: w193 -> [_ _]
                          tunnel: w192 -> [w199 w205]
                          frame #0 {
                            # "update cycle value"
                            n145 = local read "LAB03 (DISP 1)"() -> (w200:T5)
                            n146 = Unbundle By Name(w200) -> ("1 (CYCLE)"=w198:dbl)
                            n147 = case shown="True" w199 {
                              tunnel: [w202 w204] -> w197
                              tunnel: w198 -> [w202 w203]
                              frame False {
                              }
                              frame True {
                                n148 = Increment(x=w203) -> (x+1=w204:dbl)
                              }
                            }
                            n149 = Bundle By Name(cluster=w200, "1 (CYCLE)"=w197) -> (w201:T5)
                            n150 = local write "LAB03 (DISP 1)"(w201) -> ()
                          }
                          frame #1 {
                            # "stop test if test cycles reached"
                            n151 = local read "LAB03 (SETTINGS 1)"() -> (w207:T4)
                            n152 = Unbundle By Name(w207) -> ("1 (CYCLES)"=w206:dbl)
                            n153 = Greater Or Equal?(x=w211, y=w206) -> (x >= y?=w210:bool)
                            n154 = Select(t=FALSE, s=w210, f=w205) -> (s? t:f=w208:bool)
                            n155 = local write "LAB03-1 RUN"(w208) -> ()
                          }
                        }
                      }
                      frame #5 {
                        # "LAB03-2"
                        n156 = stacked-sequence {
                          seq-local: [w218 _] -> [_ w232]
                          tunnel: w217 -> [_ _]
                          tunnel: w216 -> [_ _]
                          tunnel: w215 -> [_ _]
                          tunnel: w214 -> [_ _]
                          tunnel: w213 -> [_ _]
                          tunnel: w212 -> [w219 w226]
                          frame #0 {
                            # "update cycle value"
                            n157 = local read "LAB03 (DISP 1)"() -> (w221:T5)
                            n158 = Unbundle By Name(w221) -> ("2 (CYCLE)"=w220:dbl)
                            n159 = case shown="True" w219 {
                              tunnel: [w223 w225] -> w218
                              tunnel: w220 -> [w223 w224]
                              frame False {
                              }
                              frame True {
                                n160 = Increment(x=w224) -> (x+1=w225:dbl)
                              }
                            }
                            n161 = Bundle By Name(cluster=w221, "2 (CYCLE)"=w218) -> (w222:T5)
                            n162 = local write "LAB03 (DISP 1)"(w222) -> ()
                          }
                          frame #1 {
                            # "stop test if test cycles reached"
                            n163 = local read "LAB03 (SETTINGS 1)"() -> (w228:T4)
                            n164 = Unbundle By Name(w228) -> ("2 (CYCLES)"=w227:dbl)
                            n165 = Greater Or Equal?(x=w232, y=w227) -> (x >= y?=w231:bool)
                            n166 = Select(t=FALSE, s=w231, f=w226) -> (s? t:f=w229:bool)
                            n167 = local write "LAB03-2 RUN"(w229) -> ()
                          }
                        }
                      }
                      frame #6 {
                        # "LAB04-1"
                        n168 = stacked-sequence {
                          seq-local: [w240 _] -> [_ w254]
                          tunnel: w239 -> [_ _]
                          tunnel: w238 -> [_ _]
                          tunnel: w237 -> [_ _]
                          tunnel: w236 -> [_ _]
                          tunnel: w235 -> [_ _]
                          tunnel: w234 -> [_ _]
                          tunnel: w233 -> [w242 w248]
                          frame #0 {
                            # "update cycle value"
                            n169 = local read "LAB04 (DISP 1)"() -> (w243:T5)
                            n170 = Unbundle By Name(w243) -> ("1 (CYCLE)"=w241:dbl)
                            n171 = case shown="True" w242 {
                              tunnel: [w245 w247] -> w240
                              tunnel: w241 -> [w245 w246]
                              frame False {
                              }
                              frame True {
                                n172 = Increment(x=w246) -> (x+1=w247:dbl)
                              }
                            }
                            n173 = Bundle By Name(cluster=w243, "1 (CYCLE)"=w240) -> (w244:T5)
                            n174 = local write "LAB04 (DISP 1)"(w244) -> ()
                          }
                          frame #1 {
                            # "stop test if test cycles reached"
                            n175 = local read "LAB04 (SETTINGS 1)"() -> (w250:T4)
                            n176 = Unbundle By Name(w250) -> ("1 (CYCLES)"=w249:dbl)
                            n177 = Greater Or Equal?(x=w254, y=w249) -> (x >= y?=w253:bool)
                            n178 = Select(t=FALSE, s=w253, f=w248) -> (s? t:f=w251:bool)
                            n179 = local write "LAB04-1 RUN"(w251) -> ()
                          }
                        }
                      }
                      frame #7 {
                        # "LAB04-2"
                        n180 = stacked-sequence {
                          seq-local: [w263 _] -> [_ w277]
                          tunnel: w262 -> [_ _]
                          tunnel: w261 -> [_ _]
                          tunnel: w260 -> [_ _]
                          tunnel: w259 -> [_ _]
                          tunnel: w258 -> [_ _]
                          tunnel: w257 -> [_ _]
                          tunnel: w256 -> [_ _]
                          tunnel: w255 -> [w265 w271]
                          frame #0 {
                            # "update cycle value"
                            n181 = local read "LAB04 (DISP 1)"() -> (w266:T5)
                            n182 = Unbundle By Name(w266) -> ("2 (CYCLE)"=w264:dbl)
                            n183 = case shown="True" w265 {
                              tunnel: [w268 w270] -> w263
                              tunnel: w264 -> [w268 w269]
                              frame False {
                              }
                              frame True {
                                n184 = Increment(x=w269) -> (x+1=w270:dbl)
                              }
                            }
                            n185 = Bundle By Name(cluster=w266, "2 (CYCLE)"=w263) -> (w267:T5)
                            n186 = local write "LAB04 (DISP 1)"(w267) -> ()
                          }
                          frame #1 {
                            # "stop test if test cycles reached"
                            n187 = local read "LAB04 (SETTINGS 1)"() -> (w273:T4)
                            n188 = Unbundle By Name(w273) -> ("2 (CYCLES)"=w272:dbl)
                            n189 = Greater Or Equal?(x=w277, y=w272) -> (x >= y?=w276:bool)
                            n190 = Select(t=FALSE, s=w276, f=w271) -> (s? t:f=w274:bool)
                            n191 = local write "LAB04-2 RUN"(w274) -> ()
                          }
                        }
                      }
                      frame #8 {
                        # "LAB05-1"
                        n192 = stacked-sequence {
                          seq-local: [w288 _] -> [_ w301]
                          tunnel: w286 -> [_ _]
                          tunnel: w285 -> [_ _]
                          tunnel: w284 -> [_ _]
                          tunnel: w283 -> [_ _]
                          tunnel: w282 -> [_ _]
                          tunnel: w281 -> [_ _]
                          tunnel: w280 -> [_ _]
                          tunnel: w279 -> [_ _]
                          tunnel: w278 -> [w287 w296]
                          frame #0 {
                            # "update cycle value"
                            n193 = local read "LAB05 (DISP 1)"() -> (w290:T5)
                            n194 = Unbundle By Name(w290) -> ("1 (CYCLE)"=w289:dbl)
                            n195 = case shown="True" w287 {
                              tunnel: [w292 w294] -> w288
                              tunnel: w289 -> [w292 w293]
                              frame False {
                              }
                              frame True {
                                n196 = Increment(x=w293) -> (x+1=w294:dbl)
                              }
                            }
                            n197 = Bundle By Name(cluster=w290, "1 (CYCLE)"=w288) -> (w291:T5)
                            n198 = local write "LAB05 (DISP 1)"(w291) -> ()
                          }
                          frame #1 {
                            # "stop test if test cycles reached"
                            n199 = local read "LAB05 (SETTINGS 1)"() -> (w297:T4)
                            n200 = Unbundle By Name(w297) -> ("1 (CYCLES)"=w295:dbl)
                            n201 = Greater Or Equal?(x=w301, y=w295) -> (x >= y?=w300:bool)
                            n202 = Select(t=FALSE, s=w300, f=w296) -> (s? t:f=w298:bool)
                            n203 = local write "LAB05-1 RUN"(w298) -> ()
                          }
                        }
                      }
                      frame #9 {
                        # "LAB05-2"
                        n204 = stacked-sequence {
                          seq-local: [w312 _] -> [_ w326]
                          tunnel: w311 -> [_ _]
                          tunnel: w310 -> [_ _]
                          tunnel: w309 -> [_ _]
                          tunnel: w308 -> [_ _]
                          tunnel: w307 -> [_ _]
                          tunnel: w306 -> [_ _]
                          tunnel: w305 -> [_ _]
                          tunnel: w304 -> [_ _]
                          tunnel: w303 -> [_ _]
                          tunnel: w302 -> [w313 w320]
                          frame #0 {
                            # "update cycle value"
                            n205 = local read "LAB05 (DISP 1)"() -> (w315:T5)
                            n206 = Unbundle By Name(w315) -> ("2 (CYCLE)"=w314:dbl)
                            n207 = case shown="True" w313 {
                              tunnel: [w317 w319] -> w312
                              tunnel: w314 -> [w317 w318]
                              frame False {
                              }
                              frame True {
                                n208 = Increment(x=w318) -> (x+1=w319:dbl)
                              }
                            }
                            n209 = Bundle By Name(cluster=w315, "2 (CYCLE)"=w312) -> (w316:T5)
                            n210 = local write "LAB05 (DISP 1)"(w316) -> ()
                          }
                          frame #1 {
                            # "stop test if test cycles reached"
                            n211 = local read "LAB05 (SETTINGS 1)"() -> (w322:T4)
                            n212 = Unbundle By Name(w322) -> ("2 (CYCLES)"=w321:dbl)
                            n213 = Greater Or Equal?(x=w326, y=w321) -> (x >= y?=w325:bool)
                            n214 = Select(t=FALSE, s=w325, f=w320) -> (s? t:f=w323:bool)
                            n215 = local write "LAB05-2 RUN"(w323) -> ()
                          }
                        }
                      }
                    }
                  }
                }
                n216 = local write "jig cycle"(0) -> ()
              }
            }
          }
          frame #2 {
            # "disable functions"
            n217 = stacked-sequence {
              tunnel: w336 -> [w341 _ w396]
              tunnel: w335 -> [w340 _ w395]
              tunnel: w334 -> [w339 _ w394]
              tunnel: w333 -> [w338 _ w393]
              tunnel: w332 -> [w337 _ w392]
              tunnel: w331 -> [_ w361 w391]
              tunnel: w330 -> [_ w360 w390]
              tunnel: w329 -> [_ w359 w389]
              tunnel: w328 -> [_ w358 w388]
              tunnel: w327 -> [_ w357 w387]
              frame #0 {
                n218 = Select(t=2, s=w338, f=0) -> (s? t:f=w345:i32)
                n219 = Select(t=2, s=w339, f=0) -> (s? t:f=w348:i32)
                n220 = Select(t=2, s=w337, f=0) -> (s? t:f=w342:i32)
                n221 = Select(t=2, s=w341, f=0) -> (s? t:f=w354:i32)
                n222 = Select(t=2, s=w340, f=0) -> (s? t:f=w351:i32)
                n223 = property on="LAB02-2 SELECT" class="RadioBtnsControl (strict)"("DisabledEnum"=w345) -> ()  [unwired: 2 in, 2 out]
                n224 = property on="LAB02-1 SELECT" class="RadioBtnsControl (strict)"("DisabledEnum"=w348) -> ()  [unwired: 2 in, 2 out]
                n225 = property on="LAB03-1 SELECT" class="RadioBtnsControl (strict)"("DisabledEnum"=w342) -> ()  [unwired: 2 in, 2 out]
                n226 = property on="LAB01-1 SELECT" class="RadioBtnsControl (strict)"("DisabledEnum"=w354) -> ()  [unwired: 2 in, 2 out]
                n227 = property on="LAB01-2 SELECT" class="RadioBtnsControl (strict)"("DisabledEnum"=w351) -> ()  [unwired: 2 in, 2 out]
              }
              frame #1 {
                n228 = Select(t=2, s=w357, f=0) -> (s? t:f=w362:i32)
                n229 = Select(t=2, s=w358, f=0) -> (s? t:f=w365:i32)
                n230 = Select(t=2, s=w361, f=0) -> (s? t:f=w374:i32)
                n231 = Select(t=2, s=w360, f=0) -> (s? t:f=w371:i32)
                n232 = Select(t=2, s=w359, f=0) -> (s? t:f=w368:i32)
                n233 = property on="LAB05-2 SELECT" class="RadioBtnsControl (strict)"("DisabledEnum"=w362) -> ()  [unwired: 2 in, 2 out]
                n234 = property on="LAB05-1 SELECT" class="RadioBtnsControl (strict)"("DisabledEnum"=w365) -> ()  [unwired: 2 in, 2 out]
                n235 = property on="LAB03-2 SELECT" class="RadioBtnsControl (strict)"("DisabledEnum"=w374) -> ()  [unwired: 2 in, 2 out]
                n236 = property on="LAB04-1 SELECT" class="RadioBtnsControl (strict)"("DisabledEnum"=w371) -> ()  [unwired: 2 in, 2 out]
                n237 = property on="LAB04-2 SELECT" class="RadioBtnsControl (strict)"("DisabledEnum"=w368) -> ()  [unwired: 2 in, 2 out]
              }
              frame #2 {
                # "disable calibrate if any test running"
                n238 = Or(x=w388, y=w387) -> (x .or. y?=w381:bool)
                n239 = Or(x=w390, y=w389) -> (x .or. y?=w383:bool)
                n240 = Or(x=w394, y=w393) -> (x .or. y?=w385:bool)
                n241 = Or(x=w392, y=w391) -> (x .or. y?=w384:bool)
                n242 = Or(x=w396, y=w395) -> (x .or. y?=w386:bool)
                n243 = Or(x=w384, y=w383) -> (x .or. y?=w382:bool)
                n244 = Or(x=w386, y=w385) -> (x .or. y?=w380:bool)
                n245 = Or(x=w382, y=w381) -> (x .or. y?=w379:bool)
                n246 = Or(x=w380, y=w379) -> (x .or. y?=w378:bool)
                n247 = case shown="True" w378 {
                  tunnel: [0 2] -> w377
                  frame False {
                  }
                  frame True {
                  }
                }
                n248 = property on="CALIBRATE" class="Bool (strict)"("DisabledEnum"=w377) -> ()  [unwired: 2 in, 2 out]
              }
            }
          }
          frame #3 {
            # "run calibration routine"
            n249 = local read "CALIBRATE"() -> (w399:bool)
            n250 = case shown="True" w399 {
              frame False {
              }
              frame True {
                n251 = stacked-sequence {
                  seq-local: [w400 _ _] -> [_ w402 _]
                  frame #0 {
                    n252 = call "CALIBRATION PASSWORD"() -> ("PASSWORD"=w400:string)  [unwired: 17 in, 2 out]
                  }
                  frame #1 {
                    n253 = Equal?(x=w402, y="7777") -> (x = y?=w401:bool)
                    n254 = case shown="True" w401 {
                      frame False {
                      }
                      frame True {
                        n255 = stacked-sequence {
                          frame #0 {
                            n256 = call "sub vi - calibration v1.vi"() -> ()  [unwired: 12 in]
                          }
                          frame #1 {
                            n257 = call "sub vi - get calibration values v1.vi"() -> ("LAB01 (CAL)"=w408:T8, "LAB02 (CAL)"=w407:T9, "LAB03 (CAL)"=w406:T8, "LAB04 (CAL)"=w405:T8, "calibration file error out"=w409:errorcluster, "LAB05 (CAL)"=w404:T8)  [unwired: 10 in]
                            n258 = local write "calibration file error out"(w409) -> ()
                            n259 = local write "LAB04 (CAL)"(w405) -> ()
                            n260 = local write "LAB05 (CAL)"(w404) -> ()
                            n261 = local write "LAB01 (CAL)"(w408) -> ()
                            n262 = local write "LAB02 (CAL)"(w407) -> ()
                            n263 = local write "LAB03 (CAL)"(w406) -> ()
                          }
                        }
                      }
                    }
                  }
                  frame #2 {
                    n264 = local write "CALIBRATE"(FALSE) -> ()
                  }
                }
              }
            }
          }
          frame #4 {
            # "open test files"
            n265 = Get Date/Time In Seconds() -> (seconds since 1Jan1904=w415:timestamp)
            n266 = Format Date/Time String(time format string (%c)="%Y%m%d", seconds (now)=w415) -> (date/time string=w416:string)  [unwired: 1 in]
            n267 = Format Date/Time String(time format string (%c)="%H%M", seconds (now)=w415) -> (date/time string=w413:string)  [unwired: 1 in]
            n268 = event shown="[1] \"LAB01-1RUN\": Value Change" {
              selector: _ -> [_ _]
              dyn-events: _ -> [_ _]
              timeout: 10 -> [_ _]
              tunnel: "c:\\crabtree\\Test Data\\" -> [_ w424]
              tunnel: w416 -> [_ w423]
              tunnel: w413 -> [_ w421]
              tunnel: w412 -> [_ w422]
              tunnel: w411 -> [_ w420]
              event Timeout {
                n269 = event-data() -> ()  [unwired: 1 in, 3 out]
              }
              event "LAB01-1RUN": Value Change {
                n270 = event-data() -> ()  [unwired: 1 in, 6 out]
                n271 = stacked-sequence {
                  seq-local: [w425 _ _] -> [_ w440 _]
                  tunnel: w424 -> [w436 _ _]
                  tunnel: w423 -> [w434 _ _]
                  tunnel: w422 -> [w433 _ _]
                  tunnel: w421 -> [w428 _ _]
                  tunnel: w420 -> [_ w441 _]
                  frame #0 {
                    n272 = case shown="\"TEST SET UP\", Default" w433 {
                      tunnel: ["TEST SET UP-" "CYCLE TEST-" "T-RISE TEST-"] -> w429
                      frame "TEST SET UP", Default {
                      }
                      frame "CYCLE TEST" {
                      }
                      frame "T-RISE TEST" {
                      }
                    }
                    n273 = Concatenate Strings(w436, "LAB01-1\\", w434, "\\") -> (w430:string)
                    n274 = String To Path(string=w430) -> (path=w432:path)
                    n275 = Concatenate Strings(w430, w429, w428, ".tdms") -> (w425:string)
                    n276 = Create Folder(path (use dialog)=w432) -> (error out=w431:errorcluster)  [unwired: 2 in, 2 out]
                    n277 = call <vilib>:"Clear Errors.vi"("error in (no error)"=w431) -> ()  [unwired: 6 in, 1 out]
                  }
                  frame #1 {
                    n278 = case shown="True" w441 {
                      tunnel: w440 -> [_ w442]
                      frame False {
                      }
                      frame True {
                        n279 = String To Path(string=w442) -> (path=w443:path)
                        n280 = TDMS Open(5:FALSE, 6:FALSE, 10:T13."create or replace" ("operation (0:open)"), 11:w443) -> (0:w445:errorcluster, 3:→"LAB01-1 (TDMS)":refnum<k34>)  [unwired: 3 in]
                        n281 = local write "data file error"(w445) -> ()
                      }
                    }
                  }
                  frame #2 {
                    n282 = local read "LAB01 (SETTINGS 1)"() -> (w464:T4)
                    n283 = local read "LAB01-1 (TDMS)"() -> (w465:refnum<k34>)
                    n284 = Build Array("Testers Name", "Description", "Set Test Cycles", "T-Rise minutes", "T-Rise Deg C") -> (w449:string[])
                    n285 = Unbundle By Name(w464) -> ("1 Name"=w460:string, "1 Description"=w459:string, "1 (CYCLES)"=w463:dbl, "1 (T-RISE mins)"=w462:dbl, "1 (T-RISE deg C)"=w461:dbl)
                    n286 = Number To Decimal String(number=w463) -> (decimal integer string=w458:string)  [unwired: 1 in]
                    n287 = Number To Decimal String(number=w462) -> (decimal integer string=w457:string)  [unwired: 1 in]
                    n288 = Number To Decimal String(number=w461) -> (decimal integer string=w456:string)  [unwired: 1 in]
                    n289 = Build Array(w460, w459, w458, w457, w456) -> (w455:string[])
                    n290 = TDMS Set Properties(5:w455, 7:w449, 11:w465) -> ()  [unwired: 3 in, 4 out]
                  }
                }
              }
            }
          }
          frame #5 {
            # "close test files"
            n291 = stacked-sequence {
              tunnel: w466 -> [w467]
              frame #0 {
                n292 = case shown="False" w467 {
                  frame False {
                    n293 = local read "LAB01-1 (TDMS)"() -> (w469:refnum<k34>)
                    n294 = TDMS Close(11:w469) -> (0:w468:errorcluster)  [unwired: 1 in, 1 out]
                    n295 = local write "data file error"(w468) -> ()
                  }
                  frame True {
                  }
                }
              }
            }
          }
          frame #6 {
            # "drive jigs"
            n296 = stacked-sequence {
              frame #0 {
                # "jig on"
                n297 = local read "jig cycle"() -> (w470:dbl)
                n298 = Equal?(x=w470, y=0) -> (x = y?=w472:bool)
                n299 = case shown="True" w472 {
                  frame False {
                  }
                  frame True {
                    n300 = local read "LAB01-1RUN"() -> (w473:bool)
                    n301 = local read "LAB01-2 RUN"() -> (w474:bool)
                    n302 = local read "LAB03-1 RUN"() -> (w480:bool)
                    n303 = local read "LAB03-2 RUN"() -> (w479:bool)
                    n304 = local read "LAB02-1 RUN"() -> (w482:bool)
                    n305 = local read "LAB02-2 RUN"() -> (w481:bool)
                    n306 = local read "LAB04-1 RUN"() -> (w478:bool)
                    n307 = local read "LAB04-2 RUN"() -> (w477:bool)
                    n308 = local read "LAB05-1 RUN"() -> (w476:bool)
                    n309 = local read "LAB05-2 RUN"() -> (w475:bool)
                    n310 = local write "LAB05-1 (JIG)"(w476) -> ()
                    n311 = local write "LAB05-2 (JIG)"(w475) -> ()
                    n312 = local write "LAB04-2 (JIG)"(w477) -> ()
                    n313 = local write "LAB02-1 (JIG)"(w482) -> ()
                    n314 = local write "LAB03-1 (JIG)"(w480) -> ()
                    n315 = local write "LAB04-1 (JIG)"(w478) -> ()
                    n316 = local write "LAB03-2 (JIG)"(w479) -> ()
                    n317 = local write "LAB02-2 (JIG)"(w481) -> ()
                    n318 = local write "LAB01-1 (JIG)"(w473) -> ()
                    n319 = local write "LAB01-2 (JIG)"(w474) -> ()
                  }
                }
              }
              frame #1 {
                # "jig off"
                n320 = local read "jig cycle"() -> (w485:dbl)
                n321 = local read "on loops"() -> (w484:dbl)
                n322 = Equal?(x=w485, y=w484) -> (x = y?=w483:bool)
                n323 = case shown="True" w483 {
                  frame False {
                  }
                  frame True {
                    w536 = FALSE
                    w537 = TRUE
                    w535 = 2
                    n324 = local read "LAB05-2 SELECT"() -> (w526:T3)
                    n325 = local read "LAB04-2 SELECT"() -> (w528:T3)
                    n326 = local read "LAB04-1 SELECT"() -> (w529:T3)
                    n327 = local read "LAB05-1 SELECT"() -> (w527:T3)
                    n328 = local read "LAB03-2 SELECT"() -> (w530:T3)
                    n329 = local read "LAB02-1 SELECT"() -> (w533:T3)
                    n330 = local read "LAB03-1 SELECT"() -> (w531:T3)
                    n331 = local read "LAB02-2 SELECT"() -> (w532:T3)
                    n332 = local read "LAB01-2 SELECT"() -> (w534:T3)
                    n333 = local read "LAB05-1 RUN"() -> (w496:bool)
                    n334 = local read "LAB05-2 RUN"() -> (w495:bool)
                    n335 = local read "LAB04-2 RUN"() -> (w497:bool)
                    n336 = local read "LAB04-1 RUN"() -> (w498:bool)
                    n337 = local read "LAB01-2 RUN"() -> (w503:bool)
                    n338 = local read "LAB03-2 RUN"() -> (w499:bool)
                    n339 = local read "LAB01-1RUN"() -> (w514:bool)
                    n340 = local read "LAB01-1 SELECT"() -> (w538:T3)
                    n341 = local read "LAB03-1 RUN"() -> (w500:bool)
                    n342 = local read "LAB02-1 RUN"() -> (w502:bool)
                    n343 = local read "LAB02-2 RUN"() -> (w501:bool)
                    n344 = Equal?(x=w535, y=w531) -> (x = y?=w509:bool)
                    n345 = Equal?(x=w535, y=w530) -> (x = y?=w508:bool)
                    n346 = Equal?(x=w535, y=w529) -> (x = y?=w507:bool)
                    n347 = Equal?(x=w535, y=w528) -> (x = y?=w506:bool)
                    n348 = Equal?(x=w535, y=w527) -> (x = y?=w505:bool)
                    n349 = Equal?(x=w535, y=w526) -> (x = y?=w504:bool)
                    n350 = Equal?(x=w535, y=w538) -> (x = y?=w515:bool)
                    n351 = Equal?(x=w535, y=w533) -> (x = y?=w511:bool)
                    n352 = Equal?(x=w535, y=w532) -> (x = y?=w510:bool)
                    n353 = Equal?(x=w535, y=w534) -> (x = y?=w512:bool)
                    n354 = And(x=w506, y=w497) -> (x .and. y?=w488:bool)
                    n355 = And(x=w509, y=w500) -> (x .and. y?=w491:bool)
                    n356 = And(x=w507, y=w498) -> (x .and. y?=w489:bool)
                    n357 = And(x=w504, y=w495) -> (x .and. y?=w486:bool)
                    n358 = And(x=w510, y=w501) -> (x .and. y?=w492:bool)
                    n359 = And(x=w508, y=w499) -> (x .and. y?=w490:bool)
                    n360 = And(x=w505, y=w496) -> (x .and. y?=w487:bool)
                    n361 = And(x=w512, y=w503) -> (x .and. y?=w494:bool)
                    n362 = And(x=w515, y=w514) -> (x .and. y?=w513:bool)
                    n363 = And(x=w511, y=w502) -> (x .and. y?=w493:bool)
                    n364 = Select(t=w537, s=w513, f=w536) -> (s? t:f=w516:bool)
                    n365 = Select(t=w537, s=w494, f=w536) -> (s? t:f=w517:bool)
                    n366 = Select(t=w537, s=w493, f=w536) -> (s? t:f=w518:bool)
                    n367 = Select(t=w537, s=w492, f=w536) -> (s? t:f=w519:bool)
                    n368 = Select(t=w537, s=w491, f=w536) -> (s? t:f=w520:bool)
                    n369 = Select(t=w537, s=w490, f=w536) -> (s? t:f=w521:bool)
                    n370 = Select(t=w537, s=w489, f=w536) -> (s? t:f=w522:bool)
                    n371 = Select(t=w537, s=w488, f=w536) -> (s? t:f=w523:bool)
                    n372 = Select(t=w537, s=w487, f=w536) -> (s? t:f=w524:bool)
                    n373 = Select(t=w537, s=w486, f=w536) -> (s? t:f=w525:bool)
                    n374 = local write "LAB03-2 (JIG)"(w521) -> ()
                    n375 = local write "LAB02-1 (JIG)"(w518) -> ()
                    n376 = local write "LAB02-2 (JIG)"(w519) -> ()
                    n377 = local write "LAB01-2 (JIG)"(w517) -> ()
                    n378 = local write "LAB03-1 (JIG)"(w520) -> ()
                    n379 = local write "LAB01-1 (JIG)"(w516) -> ()
                    n380 = local write "LAB05-2 (JIG)"(w525) -> ()
                    n381 = local write "LAB04-1 (JIG)"(w522) -> ()
                    n382 = local write "LAB05-1 (JIG)"(w524) -> ()
                    n383 = local write "LAB04-2 (JIG)"(w523) -> ()
                  }
                }
              }
            }
          }
          frame #7 {
            # "drive digital output"
            n384 = local read "LAB05-2 (O/I)"() -> (w544:bool)
            n385 = local read "LAB05-2 (JIG)"() -> (w543:bool)
            n386 = local read "LAB05-1 (O/I)"() -> (w546:bool)
            n387 = local read "LAB05-1 (JIG)"() -> (w545:bool)
            n388 = local read "LAB04-2 (O/I)"() -> (w548:bool)
            n389 = local read "LAB04-2 (JIG)"() -> (w547:bool)
            n390 = local read "LAB03-1 (O/I)"() -> (w553:bool)
            n391 = local read "LAB04-1 (O/I)"() -> (w549:bool)
            n392 = local read "LAB04-1 (JIG)"() -> (w542:bool)
            n393 = local read "LAB02-1 (O/I)"() -> (w557:bool)
            n394 = local read "LAB02-2 (O/I)"() -> (w555:bool)
            n395 = local read "LAB03-2 (O/I)"() -> (w551:bool)
            n396 = local read "LAB03-2 (JIG)"() -> (w550:bool)
            n397 = local read "LAB02-1 (JIG)"() -> (w556:bool)
            n398 = local read "LAB02-2 (JIG)"() -> (w554:bool)
            n399 = local read "LAB03-1 (JIG)"() -> (w552:bool)
            n400 = local read "LAB01-2 (O/I)"() -> (w559:bool)
            n401 = local read "LAB01-2 (JIG)"() -> (w558:bool)
            n402 = local read "LAB01-1 (O/I)"() -> (w561:bool)
            n403 = local read "LAB01-1 (JIG)"() -> (w560:bool)
            n404 = Build Array(w548, w547, w546, w545, w544, w543) -> (w539:bool[])
            n405 = Build Array(w554, w553, w552, w551, w550, w549, w542) -> (w540:bool[])
            n406 = Build Array(w561, w560, w559, w558, w557, w556, w555) -> (w541:bool[])
            n407 = call "sub vi - Drive Relays All v6.vi"("Array #2"=w539, "Array #1"=w540, "Array #0"=w541) -> ()  [unwired: 8 in, 1 out]
          }
          frame #8 {
            # "get temperature values"
            n408 = stacked-sequence {
              frame #0 {
                n409 = local read "jig cycle"() -> (w562:dbl)
                n410 = local read "on loops"() -> (w565:dbl)
                n411 = local read "jig cycle"() -> (w567:dbl)
                n412 = Add(x=w565, y=1) -> (x+y=w566:dbl)
                n413 = Equal?(x=w567, y=0) -> (x = y?=w568:bool)
                n414 = Equal?(x=w562, y=w566) -> (x = y?=w563:bool)
                n415 = case shown="True" w568 {
                  frame False {
                  }
                  frame True {
                    w580 = FALSE
                    w581 = TRUE
                    n416 = local write "TEMP update"(TRUE) -> ()
                    n417 = call "sub vi - GET ALL TEMP v3.vi"("LA01-EN"=w581, "LA02-EN"=w581, "LA03-EN"=w581, "LA04-EN"=w580, "LA05-EN"=w580, "Gen Cal Value"=1.0) -> ("LA01 TEMP"=w579:T14, "LA02 TEMP"=w577:T14, "LA03 TEMP"=w576:T14)  [unwired: 4 in, 3 out]
                    n418 = local write "LAB03 TEMP"(w576) -> ()
                    n419 = local write "LAB02 TEMP"(w577) -> ()
                    n420 = local write "LAB01 TEMP"(w579) -> ()
                  }
                }
                n421 = case shown="True" w563 {
                  frame False {
                  }
                  frame True {
                    w573 = TRUE
                    w574 = FALSE
                    n422 = local write "TEMP update"(TRUE) -> ()
                    n423 = call "sub vi - GET ALL TEMP v3.vi"("LA01-EN"=w574, "LA02-EN"=w574, "LA03-EN"=w574, "LA04-EN"=w573, "LA05-EN"=w573, "Gen Cal Value"=1.0) -> ("LA04 TEMP"=w571:T14, "LA05 TEMP"=w570:T14)  [unwired: 4 in, 4 out]
                    n424 = local write "LAB04 TEMP"(w571) -> ()
                    n425 = local write "LAB05 TEMP"(w570) -> ()
                  }
                }
              }
              frame #1 {
                n426 = local read "LAB01 (CAL)"() -> (w599:T8)
                n427 = local read "LAB01 TEMP"() -> (w600:T7)
                n428 = Unbundle By Name(w600) -> ("T1 Live"=w590:dbl, "T1 Neut"=w589:dbl, "T2 Live"=w588:dbl, "T2 Neut"=w587:dbl)  [unwired: 2 out]
                n429 = Unbundle By Name(w599) -> ("1 (TL) cal"=w586:dbl, "1 (TN) cal"=w585:dbl, "2 (TL) cal"=w584:dbl, "2 (TN) cal"=w583:dbl)  [unwired: 6 out]
                n430 = Multiply(x=w590, y=w586) -> (x*y=w596:dbl)
                n431 = Multiply(x=w589, y=w585) -> (x*y=w595:dbl)
                n432 = Multiply(x=w588, y=w584) -> (x*y=w592:dbl)
                n433 = Multiply(x=w587, y=w583) -> (x*y=w591:dbl)
                n434 = local read "LAB01-2 (SIG)"() -> (w594:T2)
                n435 = local read "LAB01-1 (SIG)"() -> (w598:T2)
                n436 = Bundle By Name(cluster=w598, "Tmp Live"=w596, "Tmp Neut"=w595) -> (w597:T2)
                n437 = Bundle By Name(cluster=w594, "Tmp Live"=w592, "Tmp Neut"=w591) -> (w593:T2)
                n438 = local write "LAB01-1 (SIG)"(w597) -> ()
                n439 = local write "LAB01-2 (SIG)"(w593) -> ()
              }
              frame #2 {
                n440 = local read "LAB02 (CAL)"() -> (w617:T9)
                n441 = local read "LAB02 TEMP"() -> (w618:T7)
                n442 = Unbundle By Name(w618) -> ("T1 Live"=w608:dbl, "T1 Neut"=w607:dbl, "T2 Live"=w606:dbl, "T2 Neut"=w605:dbl)  [unwired: 2 out]
                n443 = Unbundle By Name(w617) -> ("1 (TL) cal"=w604:dbl, "1 (TN) cal"=w603:dbl, "2 (TL) cal"=w602:dbl, "2 (TN) cal"=w601:dbl)  [unwired: 6 out]
                n444 = Multiply(x=w608, y=w604) -> (x*y=w614:dbl)
                n445 = Multiply(x=w607, y=w603) -> (x*y=w613:dbl)
                n446 = Multiply(x=w606, y=w602) -> (x*y=w610:dbl)
                n447 = Multiply(x=w605, y=w601) -> (x*y=w609:dbl)
                n448 = local read "LAB02-2 (SIG)"() -> (w612:T2)
                n449 = local read "LAB02-1 (SIG)"() -> (w616:T2)
                n450 = Bundle By Name(cluster=w616, "Tmp Live"=w614, "Tmp Neut"=w613) -> (w615:T2)
                n451 = Bundle By Name(cluster=w612, "Tmp Live"=w610, "Tmp Neut"=w609) -> (w611:T2)
                n452 = local write "LAB02-1 (SIG)"(w615) -> ()
                n453 = local write "LAB02-2 (SIG)"(w611) -> ()
              }
              frame #3 {
                n454 = local read "LAB03 (CAL)"() -> (w635:T8)
                n455 = local read "LAB03 TEMP"() -> (w636:T7)
                n456 = Unbundle By Name(w636) -> ("T1 Live"=w626:dbl, "T1 Neut"=w625:dbl, "T2 Live"=w624:dbl, "T2 Neut"=w623:dbl)  [unwired: 2 out]
                n457 = Unbundle By Name(w635) -> ("1 (TL) cal"=w622:dbl, "1 (TN) cal"=w621:dbl, "2 (TL) cal"=w620:dbl, "2 (TN) cal"=w619:dbl)  [unwired: 6 out]
                n458 = Multiply(x=w626, y=w622) -> (x*y=w632:dbl)
                n459 = Multiply(x=w625, y=w621) -> (x*y=w631:dbl)
                n460 = Multiply(x=w624, y=w620) -> (x*y=w628:dbl)
                n461 = Multiply(x=w623, y=w619) -> (x*y=w627:dbl)
                n462 = local read "LAB03-2 (SIG)"() -> (w630:T2)
                n463 = local read "LAB03-1 (SIG)"() -> (w634:T2)
                n464 = Bundle By Name(cluster=w634, "Tmp Live"=w632, "Tmp Neut"=w631) -> (w633:T2)
                n465 = Bundle By Name(cluster=w630, "Tmp Live"=w628, "Tmp Neut"=w627) -> (w629:T2)
                n466 = local write "LAB03-1 (SIG)"(w633) -> ()
                n467 = local write "LAB03-2 (SIG)"(w629) -> ()
              }
              frame #4 {
                n468 = local read "LAB04 (CAL)"() -> (w653:T8)
                n469 = local read "LAB04 TEMP"() -> (w654:T7)
                n470 = Unbundle By Name(w654) -> ("T1 Live"=w644:dbl, "T1 Neut"=w643:dbl, "T2 Live"=w642:dbl, "T2 Neut"=w641:dbl)  [unwired: 2 out]
                n471 = Unbundle By Name(w653) -> ("1 (TL) cal"=w640:dbl, "1 (TN) cal"=w639:dbl, "2 (TL) cal"=w638:dbl, "2 (TN) cal"=w637:dbl)  [unwired: 6 out]
                n472 = Multiply(x=w644, y=w640) -> (x*y=w650:dbl)
                n473 = Multiply(x=w643, y=w639) -> (x*y=w649:dbl)
                n474 = Multiply(x=w642, y=w638) -> (x*y=w646:dbl)
                n475 = Multiply(x=w641, y=w637) -> (x*y=w645:dbl)
                n476 = local read "LAB04-2 (SIG)"() -> (w648:T2)
                n477 = local read "LAB04-1 (SIG)"() -> (w652:T2)
                n478 = Bundle By Name(cluster=w652, "Tmp Live"=w650, "Tmp Neut"=w649) -> (w651:T2)
                n479 = Bundle By Name(cluster=w648, "Tmp Live"=w646, "Tmp Neut"=w645) -> (w647:T2)
                n480 = local write "LAB04-1 (SIG)"(w651) -> ()
                n481 = local write "LAB04-2 (SIG)"(w647) -> ()
              }
              frame #5 {
                n482 = local read "LAB05 (CAL)"() -> (w671:T8)
                n483 = local read "LAB05 TEMP"() -> (w672:T7)
                n484 = Unbundle By Name(w672) -> ("T1 Live"=w662:dbl, "T1 Neut"=w661:dbl, "T2 Live"=w660:dbl, "T2 Neut"=w659:dbl)  [unwired: 2 out]
                n485 = Unbundle By Name(w671) -> ("1 (TL) cal"=w658:dbl, "1 (TN) cal"=w657:dbl, "2 (TL) cal"=w656:dbl, "2 (TN) cal"=w655:dbl)  [unwired: 6 out]
                n486 = Multiply(x=w662, y=w658) -> (x*y=w668:dbl)
                n487 = Multiply(x=w661, y=w657) -> (x*y=w667:dbl)
                n488 = Multiply(x=w660, y=w656) -> (x*y=w664:dbl)
                n489 = Multiply(x=w659, y=w655) -> (x*y=w663:dbl)
                n490 = local read "LAB05-2 (SIG)"() -> (w666:T2)
                n491 = local read "LAB05-1 (SIG)"() -> (w670:T2)
                n492 = Bundle By Name(cluster=w670, "Tmp Live"=w668, "Tmp Neut"=w667) -> (w669:T2)
                n493 = Bundle By Name(cluster=w666, "Tmp Live"=w664, "Tmp Neut"=w663) -> (w665:T2)
                n494 = local write "LAB05-1 (SIG)"(w669) -> ()
                n495 = local write "LAB05-2 (SIG)"(w665) -> ()
              }
            }
          }
          frame #9 {
            # "get analog values"
            n496 = local read "on loops"() -> (w679:dbl)
            n497 = local read "jig cycle"() -> (w676:dbl)
            n498 = Add(x=w679, y=2) -> (x+y=w677:dbl)
            n499 = Equal?(x=w676, y=1) -> (x = y?=w674:bool)
            n500 = Equal?(x=w676, y=w677) -> (x = y?=w675:bool)
            n501 = Or(x=w674, y=w675) -> (x .or. y?=w673:bool)
            n502 = case shown="True" w673 {
              frame False {
              }
              frame True {
                n503 = call "sub vi - Read Analog All v7.vi"() -> ("Analog loop time"=w687:dbl, "array GRAPH"=w686:dynamicdata[], "LAB01"=w685:T15, "LAB02"=w684:T16, "LAB03"=w683:T17, "LAB04"=w682:T18, "array ERROR"=w688:errorcluster[], "LAB05"=w681:T19)  [unwired: 8 in]
                n504 = stacked-sequence {
                  tunnel: w688 -> [w691 _ _ _ _ _]
                  tunnel: w687 -> [w690 _ _ _ _ _]
                  tunnel: w686 -> [w689 _ _ _ _ _]
                  tunnel: w685 -> [_ w736 _ _ _ _]
                  tunnel: w684 -> [_ _ w737 _ _ _]
                  tunnel: w683 -> [_ _ _ w761 _ _]
                  tunnel: w682 -> [_ _ _ _ w785 _]
                  tunnel: w681 -> [_ _ _ _ _ w809]
                  frame #0 {
                    n505 = local write "AI update"(TRUE) -> ()
                    n506 = Index Array(array=w689, index=6) -> (element=→"LAB04-1 (GRAPH)":dynamicdata)
                    n507 = Index Array(array=w689, index=7) -> (element=→"LAB04-2 (GRAPH)":dynamicdata)
                    n508 = Index Array(array=w689, index=9) -> (element=→"LAB05-2 (GRAPH)":dynamicdata)
                    n509 = Index Array(array=w689, index=8) -> (element=→"LAB05-1 (GRAPH)":dynamicdata)
                    n510 = Index Array(array=w689, index=5) -> (element=→"LAB03-2 (GRAPH)":dynamicdata)
                    n511 = Index Array(array=w689, index=0) -> (element=→"LAB01-1 (GRAPH)":dynamicdata)
                    n512 = Index Array(array=w689, index=1) -> (element=→"LAB01-2 (GRAPH)":dynamicdata)
                    n513 = Index Array(array=w689, index=2) -> (element=→"LAB02-1 (GRAPH)":dynamicdata)
                    n514 = Index Array(array=w689, index=3) -> (element=→"LAB02-2 (GRAPH)":dynamicdata)
                    n515 = Index Array(array=w689, index=4) -> (element=→"LAB03-1 (GRAPH)":dynamicdata)
                    "AI loop time" <- w690
                    "Analog Error Array" <- w691
                  }
                  frame #1 {
                    n516 = local read "LAB01 (CAL)"() -> (w735:T8)
                    n517 = Unbundle By Name(w736) -> ("LAB01-1 (A)"=w734:dbl, "LAB01-1 (V)"=w733:dbl, "LAB01-1 (PF)"=w732:dbl, "LAB01-2 (A)"=w731:dbl, "LAB01-2 (V)"=w730:dbl, "LAB01-2 (PF)"=w729:dbl)
                    n518 = Unbundle By Name(w735) -> ("1  (A) cal"=w728:dbl, "1 (V) cal"=w727:dbl, "1 (PF) cal"=w726:dbl, "2 (A) cal"=w725:dbl, "2 (V) cal"=w724:dbl, "2 (PF) cal"=w723:dbl)  [unwired: 4 out]
                    n519 = Multiply(x=w734, y=w728) -> (x*y=w721:dbl)
                    n520 = Multiply(x=w733, y=w727) -> (x*y=w720:dbl)
                    n521 = Multiply(x=w732, y=w726) -> (x*y=w719:dbl)
                    n522 = Multiply(x=w731, y=w725) -> (x*y=w715:dbl)
                    n523 = local read "LAB01-1 (SIG)"() -> (w722:T2)
                    n524 = Multiply(x=w730, y=w724) -> (x*y=w714:dbl)
                    n525 = Multiply(x=w729, y=w723) -> (x*y=w713:dbl)
                    n526 = local read "LAB01-2 (SIG)"() -> (w717:T2)
                    n527 = Bundle By Name(cluster=w722, "AMPS"=w721, "VOLTS"=w720, "PF"=w719) -> (w718:T2)
                    n528 = Bundle By Name(cluster=w717, "AMPS"=w715, "VOLTS"=w714, "PF"=w713) -> (w716:T2)
                    n529 = local write "LAB01-2 (SIG)"(w716) -> ()
                    n530 = local write "LAB01-1 (SIG)"(w718) -> ()
                  }
                  frame #2 {
                    n531 = local read "LAB02 (CAL)"() -> (w760:T9)
                    n532 = Unbundle By Name(w737) -> ("LAB02-1 (A)"=w759:dbl, "LAB02-1 (V)"=w758:dbl, "LAB02-1 (PF)"=w757:dbl, "LAB02-2 (A)"=w756:dbl, "LAB02-2 (V)"=w755:dbl, "LAB02-2 (PF)"=w754:dbl)
                    n533 = Unbundle By Name(w760) -> ("1 (A) cal"=w753:dbl, "1 (V) cal"=w752:dbl, "1 (PF) cal"=w751:dbl, "2 (A) cal"=w750:dbl, "2 (V) cal"=w749:dbl, "2 (PF) cal"=w748:dbl)  [unwired: 4 out]
                    n534 = Multiply(x=w759, y=w753) -> (x*y=w746:dbl)
                    n535 = Multiply(x=w758, y=w752) -> (x*y=w745:dbl)
                    n536 = Multiply(x=w757, y=w751) -> (x*y=w744:dbl)
                    n537 = Multiply(x=w756, y=w750) -> (x*y=w740:dbl)
                    n538 = local read "LAB02-1 (SIG)"() -> (w747:T2)
                    n539 = Multiply(x=w755, y=w749) -> (x*y=w739:dbl)
                    n540 = Multiply(x=w754, y=w748) -> (x*y=w738:dbl)
                    n541 = local read "LAB02-2 (SIG)"() -> (w742:T2)
                    n542 = Bundle By Name(cluster=w747, "AMPS"=w746, "VOLTS"=w745, "PF"=w744) -> (w743:T2)
                    n543 = Bundle By Name(cluster=w742, "AMPS"=w740, "VOLTS"=w739, "PF"=w738) -> (w741:T2)
                    n544 = local write "LAB02-2 (SIG)"(w741) -> ()
                    n545 = local write "LAB02-1 (SIG)"(w743) -> ()
                  }
                  frame #3 {
                    n546 = local read "LAB03 (CAL)"() -> (w784:T8)
                    n547 = Unbundle By Name(w761) -> ("LAB03-1 (A)"=w783:dbl, "LAB03-1 (V)"=w782:dbl, "LAB03-1 (PF)"=w781:dbl, "LAB03-2 (A)"=w780:dbl, "LAB03-2 (V)"=w779:dbl, "LAB03-2 (PF)"=w778:dbl)
                    n548 = Unbundle By Name(w784) -> ("1  (A) cal"=w777:dbl, "1 (V) cal"=w776:dbl, "1 (PF) cal"=w775:dbl, "2 (A) cal"=w774:dbl, "2 (V) cal"=w773:dbl, "2 (PF) cal"=w772:dbl)  [unwired: 4 out]
                    n549 = Multiply(x=w783, y=w777) -> (x*y=w770:dbl)
                    n550 = Multiply(x=w782, y=w776) -> (x*y=w769:dbl)
                    n551 = Multiply(x=w781, y=w775) -> (x*y=w768:dbl)
                    n552 = Multiply(x=w780, y=w774) -> (x*y=w764:dbl)
                    n553 = local read "LAB03-1 (SIG)"() -> (w771:T2)
                    n554 = Multiply(x=w779, y=w773) -> (x*y=w763:dbl)
                    n555 = Multiply(x=w778, y=w772) -> (x*y=w762:dbl)
                    n556 = local read "LAB03-1 (SIG)"() -> (w766:T2)
                    n557 = Bundle By Name(cluster=w771, "AMPS"=w770, "VOLTS"=w769, "PF"=w768) -> (w767:T2)
                    n558 = Bundle By Name(cluster=w766, "AMPS"=w764, "VOLTS"=w763, "PF"=w762) -> (w765:T2)
                    n559 = local write "LAB03-1 (SIG)"(w765) -> ()
                    n560 = local write "LAB03-1 (SIG)"(w767) -> ()
                  }
                  frame #4 {
                    n561 = local read "LAB04 (CAL)"() -> (w808:T8)
                    n562 = Unbundle By Name(w785) -> ("LAB04-1 (A)"=w807:dbl, "LAB04-1 (V)"=w806:dbl, "LAB04-1 (PF)"=w805:dbl, "LAB04-2 (A)"=w804:dbl, "LAB04-2 (V)"=w803:dbl, "LAB04-2 (PF)"=w802:dbl)
                    n563 = Unbundle By Name(w808) -> ("1  (A) cal"=w801:dbl, "1 (V) cal"=w800:dbl, "1 (PF) cal"=w799:dbl, "2 (A) cal"=w798:dbl, "2 (V) cal"=w797:dbl, "2 (PF) cal"=w796:dbl)  [unwired: 4 out]
                    n564 = Multiply(x=w807, y=w801) -> (x*y=w794:dbl)
                    n565 = Multiply(x=w806, y=w800) -> (x*y=w793:dbl)
                    n566 = Multiply(x=w805, y=w799) -> (x*y=w792:dbl)
                    n567 = Multiply(x=w804, y=w798) -> (x*y=w788:dbl)
                    n568 = local read "LAB04-1 (SIG)"() -> (w795:T2)
                    n569 = Multiply(x=w803, y=w797) -> (x*y=w787:dbl)
                    n570 = Multiply(x=w802, y=w796) -> (x*y=w786:dbl)
                    n571 = local read "LAB04-2 (SIG)"() -> (w790:T2)
                    n572 = Bundle By Name(cluster=w795, "AMPS"=w794, "VOLTS"=w793, "PF"=w792) -> (w791:T2)
                    n573 = Bundle By Name(cluster=w790, "AMPS"=w788, "VOLTS"=w787, "PF"=w786) -> (w789:T2)
                    n574 = local write "LAB04-2 (SIG)"(w789) -> ()
                    n575 = local write "LAB04-1 (SIG)"(w791) -> ()
                  }
                  frame #5 {
                    n576 = local read "LAB05 (CAL)"() -> (w832:T8)
                    n577 = Unbundle By Name(w809) -> ("LAB05-1 (A)"=w831:dbl, "LAB05-1 (V)"=w830:dbl, "LAB05-1 (PF)"=w829:dbl, "LAB05-2 (A)"=w828:dbl, "LAB05-2 (V)"=w827:dbl, "LAB05-2 (PF)"=w826:dbl)
                    n578 = Unbundle By Name(w832) -> ("1  (A) cal"=w825:dbl, "1 (V) cal"=w824:dbl, "1 (PF) cal"=w823:dbl, "2 (A) cal"=w822:dbl, "2 (V) cal"=w821:dbl, "2 (PF) cal"=w820:dbl)  [unwired: 4 out]
                    n579 = Multiply(x=w831, y=w825) -> (x*y=w818:dbl)
                    n580 = Multiply(x=w830, y=w824) -> (x*y=w817:dbl)
                    n581 = Multiply(x=w829, y=w823) -> (x*y=w816:dbl)
                    n582 = Multiply(x=w828, y=w822) -> (x*y=w812:dbl)
                    n583 = local read "LAB05-1 (SIG)"() -> (w819:T2)
                    n584 = Multiply(x=w827, y=w821) -> (x*y=w811:dbl)
                    n585 = Multiply(x=w826, y=w820) -> (x*y=w810:dbl)
                    n586 = local read "LAB05-2 (SIG)"() -> (w814:T2)
                    n587 = Bundle By Name(cluster=w819, "AMPS"=w818, "VOLTS"=w817, "PF"=w816) -> (w815:T2)
                    n588 = Bundle By Name(cluster=w814, "AMPS"=w812, "VOLTS"=w811, "PF"=w810) -> (w813:T2)
                    n589 = local write "LAB05-2 (SIG)"(w813) -> ()
                    n590 = local write "LAB05-1 (SIG)"(w815) -> ()
                  }
                }
              }
            }
          }
          frame #10 {
            # "save test data to file"
            n591 = local read "on loops"() -> (w840:dbl)
            n592 = local read "jig cycle"() -> (w837:dbl)
            n593 = Add(x=w840, y=2) -> (x+y=w838:dbl)
            n594 = Equal?(x=w837, y=1) -> (x = y?=w835:bool)
            n595 = Equal?(x=w837, y=w838) -> (x = y?=w836:bool)
            n596 = Or(x=w835, y=w836) -> (x .or. y?=w834:bool)
            n597 = case shown="True" w834 {
              tunnel: w833 -> [_ w842]
              frame False {
              }
              frame True {
                n598 = stacked-sequence {
                  tunnel: w842 -> [w843]
                  frame #0 {
                    # "LAB01-1"
                    n599 = case shown="True" w843 {
                      frame False {
                      }
                      frame True {
                        n600 = local read "LAB01 (DISP 1)"() -> (w885:T5)
                        n601 = local read "LAB01-1 (SIG)"() -> (w886:T2)
                        n602 = local read "LAB01-1 (TDMS)"() -> (w887:refnum<k34>)
                        n603 = Build Array("TEMP Neut") -> (w851:string[])
                        n604 = Build Array("CYCLE") -> (w846:string[])
                        n605 = Build Array("TEMP Live") -> (w856:string[])
                        n606 = Build Array("PF") -> (w861:string[])
                        n607 = Build Array("AMPS") -> (w882:string[])
                        n608 = Build Array("VOLTS") -> (w873:string[])
                        n609 = Unbundle(w886) -> ("AMPS"=w881:dbl, "VOLTS"=w870:dbl, "PF"=w869:dbl, "Tmp Live"=w868:dbl, "Tmp Neut"=w871:dbl)
                        n610 = Unbundle(w885) -> ("1 (CYCLE)"=w866:dbl)  [unwired: 5 out]
                        n611 = Build Array(w870) -> (w867:dbl[])
                        n612 = Build Array(w869) -> (w860:dbl[])
                        n613 = Build Array(w868) -> (w855:dbl[])
                        n614 = Build Array(w871) -> (w850:dbl[])
                        n615 = Build Array(w881) -> (w880:dbl[])
                        n616 = Build Array(w866) -> (w845:dbl[])
                        n617 = TDMS Write(0:w887, 5:"LAB01-1 TEST VALUES", 7:w882, 9:w880) -> (4:w875:refnum<k34>, 6:w874:string, 15:w862:errorcluster)  [unwired: 2 in, 1 out]
                        n618 = TDMS Write(0:w875, 5:w874, 7:w873, 9:w867, 11:w862) -> (4:w865:refnum<k34>, 6:w864:string, 15:w863:errorcluster)  [unwired: 1 in, 1 out]
                        n619 = TDMS Write(0:w865, 5:w864, 7:w861, 9:w860, 11:w863) -> (4:w859:refnum<k34>, 6:w858:string, 15:w857:errorcluster)  [unwired: 1 in, 1 out]
                        n620 = TDMS Write(0:w859, 5:w858, 7:w856, 9:w855, 11:w857) -> (4:w854:refnum<k34>, 6:w853:string, 15:w852:errorcluster)  [unwired: 1 in, 1 out]
                        n621 = TDMS Write(0:w854, 5:w853, 7:w851, 9:w850, 11:w852) -> (4:w849:refnum<k34>, 6:w848:string, 15:w847:errorcluster)  [unwired: 1 in, 1 out]
                        n622 = TDMS Write(0:w849, 5:w848, 7:w846, 9:w845, 11:w847) -> (15:w844:errorcluster)  [unwired: 1 in, 3 out]
                        n623 = local write "data file error"(w844) -> ()
                      }
                    }
                  }
                }
              }
            }
          }
          frame #11 {
          }
          frame #12 {
          }
        }
        n624 = node-c288() -> ()  [unwired: 1 in, 1 out]
        "loops" <- w24
      }
      n625 = node-c288(w10) -> ()  [unwired: 1 out]
    }
  }
